vi "Main.vi"() -> ()   [LabVIEW 2019]
doc: "This template is for the Queued Message Handler design pattern.\n\nThe Event Handling Loop generates messages based on user interface actions.\n\nThe Message Handling Loop processes messages generated by the Event Handling Loop, or by other messages. The messages are string values, so new messages can be added easily to the Message Cases case structure in the Message Handling Loop. Each message cluster can also provide an optional value for Message Data, which is a variant that can be converted to whatever message-specific data is required."
uses:
  controls/UI Data.ctl
  C:/Program Files (x86)/National Instruments/LabVIEW 2019/examples/Instrument IO/Serial/support/Serial - Settings.ctl
  support/Message Queue/Enqueue Message (Single).vi
  support/Message Queue/Enqueue Message (Array).vi
  <instrlib>/Yokogawa WT300 Series/Public/Utility/Function/Create Function String (Voltage).vi
  <instrlib>/Yokogawa WT300 Series/Public/Data/Read Measurement (Normal).vi
  <instrlib>/Yokogawa WT300 Series/Public/Utility/Function/Create Function String (Current).vi
  <instrlib>/Yokogawa WT300 Series/Public/Utility/Function/Create Function String (Power).vi
  <instrlib>/Yokogawa WT300 Series/Public/Utility/Function/Create Function String (Integrate).vi
  <vilib>/Instr/_visa.llb/VISA Configure Serial Port (Instr).vi
  <vilib>/Utility/error.llb/Error Cluster From Error Code.vi
  <vilib>/ErrorRing/Error Ring.xnode
  support/Message Queue/Message Queue.lvlib
  support/User Event - Stop/User Event - Stop.lvlib
  <instrlib>/Yokogawa WT300 Series/Yokogawa WT300 Series.lvlib
  <instrlib>/Prodigit 331xF Series/Prodigit 331xF Series.lvlib
panel:
  in  "Tab Control":enum32{"General Setup", "Efficiency Test"}(tab)
  in  "AC Source Address":refnum<visa-resource-name>
  in  "Load Address":refnum<visa-resource-name>
  in  "Model Name":string
  in  "Switch":refnum<visa-resource-name>
  in  "PM Address":refnum<visa-resource-name>
  in  "Load":enum16{"ABC", "DEF", "GHI"}(ring)
  in  "Load(A)":dbl
  in  "Socket":enum16{"ABC", "DEF", "GHI"}(ring)
  in  "Input_Source[]":T1(array[ring])
  in  "Warm(s)":dbl
  out "Output_Load[]":dbl[](array[numeric])
  out "EFF":dbl format="%#_2f"
  out "P.F":dbl format="%#_2f"
  out "Counter":string
  out "V":dbl format="%#_5g"
  out "W":dbl format="%#_5g"
  out "A":dbl format="%#_5g"
  out "Function":string[](array[string])
  out "Measurement":dbl[](array[numeric])
  out "W":dbl format="%#_2f"
  out "A":dbl format="%#_2f"
  out "V":dbl format="%#_2f"
  out "Status":string
  in  "Do Something Else <Replace Me>":bool
  in  "Do Something <Replace Me>":bool
  in  "Exit":bool
  # "100%"
  # "75%"
  # "50%"
  # "25%"
  # "0%"
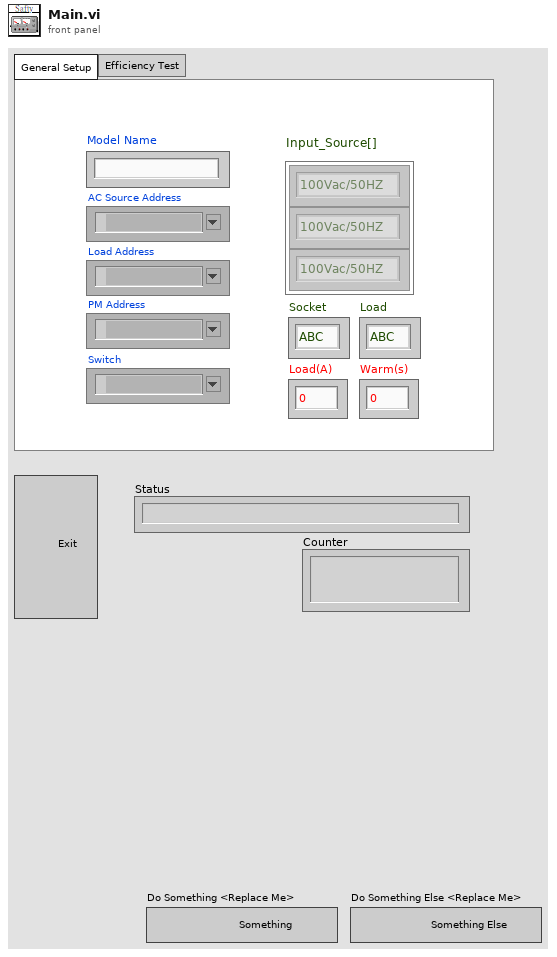
[diagram p1: front panel]
types:
  T1 = enum16{"100Vac/50HZ", "115Vac/60Hz", "230Vac/50Hz"}[]
  T2 = typedef "UI Data.ctl" = cluster{"Boolean <Replace Me>":bool, "Message":string, "Numeric <Replace Me>":dbl, "Do Something Ref":refnum<vi>, "Serial - Settings.ctlDo Something Else Ref":refnum<vi>, "Data Display Ref":refnum<vi>, "Exit Button Ref":refnum<vi>, "Model Name":string, "Input_Source[]":enum16{"100Vac/50HZ", "115Vac/60Hz", "230Vac/50Hz"}[], "RlyPort":refnum<visa-resource-name>, "ACSourcePara":cluster{"RangSelect":enum16{":SOUR:RANG LOW;", ":SOUR:RANG HIGH;", ":SOUR:RANG AUTO;"}, "Volt(V)":string, "Freq(Hz)":string, "OutpSlect":enum16{":SOUR:TURN OFF;", ":SOUR:TURN ON;"}, "TurnSlect":enum16{":SOUR:TURN OFF;", ":SOUR:TURN ON;"}}, "Step":cluster{"UI":string[], "PM":string[], "Load":string[]}, "PM Address":refnum<visa-resource-name>, "InputData":cluster{"V":dbl[], "A":dbl[], "W":dbl[], "P.F":dbl[], "EFF":dbl[], "Record":bool}, "LoadAddress":refnum<visa-resource-name>, "RLY":cluster{"Num":enum16{"AA", "01", "02", "03", "04", "05", "06", "07", "08", "09", "10", "11", "12", "13", "14", "15", "16", "17", "18", "19", "20", "21", "22", "23", "24"}, "ON/OFF":bool, "REST?":u16}, "AC Source Address":refnum<visa-resource-name>, "WarmUp Time":dbl, "Integrate Time":dbl, "Function":string[], "Measurement":dbl[], "SourceIndex":i32, "Socket":enum16{"ABC", "DEF", "GHI"}, "LoadSel":enum16{"ABC", "DEF", "GHI"}, "Load":cluster{"Current Level (F:Low)":u16, "OutputLoad[]":dbl[], "Index":i32, "Load (ON/Off)":bool, "Channel (0:Channel 1)":u16, "Value[]":cluster{"A":dbl[], "W":dbl[], "V":dbl[]}, "Record":bool}}
  T3 = typedef "Message Queue.lvlib/All Message Queues.ctl" = cluster{"UI":refnum<queue>, "PM":refnum<queue>, "Load":refnum<queue>}
  T4 = cluster{"Current Level (F:Low)":u16, "OutputLoad[]":dbl[], "Index":i32, "Load (ON/Off)":bool, "Channel (0:Channel 1)":u16, "Value[]":cluster{"A":dbl[], "W":dbl[], "V":dbl[]}, "Record":bool}
  T5 = cluster{"Current Level (F:Low)":u16, "OutputLoad[]":dbl[], "Index":i32, "Load (ON/Off)":bool, "Channel (0:Channel 1)":u16, "Value[]":cluster{"A":dbl[], "W":dbl[], "V":dbl[]}, "Record":bool}[]
  T6 = cluster{"V":dbl[], "A":dbl[], "W":dbl[], "P.F":dbl[], "EFF":dbl[], "Record":bool}
  T7 = typedef "Serial - Settings.ctl" = cluster{"baud rate":u32, "data bits":u16, "parity":enum16{"None", "Odd", "Even", "Mark", "Space"}, "stop bits":u16, "flow control":u16}
  T8 = enum16{":SOUR:RANG LOW;", ":SOUR:RANG HIGH;", ":SOUR:RANG AUTO;"}
  T9 = enum16{"SetRange", "SetVoltage", "SetFreq", "OUTP", "TurnOn"}
  T10 = enum16{"AA", "01", "02", "03", "04", "05", "06", "07", "08", "09", "10", "11", "12", "13", "14", "15", "16", "17", "18", "19", "20", "21", "22", "23", "24"}
  T11 = enum16{"100Vac/50HZ", "115Vac/60Hz", "230Vac/50Hz"}
  T12 = cluster{"RangSelect":enum16{":SOUR:RANG LOW;", ":SOUR:RANG HIGH;", ":SOUR:RANG AUTO;"}, "Volt(V)":string, "Freq(Hz)":string, "OutpSlect":enum16{":SOUR:TURN OFF;", ":SOUR:TURN ON;"}, "TurnSlect":enum16{":SOUR:TURN OFF;", ":SOUR:TURN ON;"}}
  T13 = cluster{"Num":enum16{"AA", "01", "02", "03", "04", "05", "06", "07", "08", "09", "10", "11", "12", "13", "14", "15", "16", "17", "18", "19", "20", "21", "22", "23", "24"}, "ON/OFF":bool, "REST?":u16}
  T14 = cluster{"V":dbl[], "A":dbl[], "W":dbl[], "P.F":dbl[], "EFF":dbl[], "Record":bool}[]
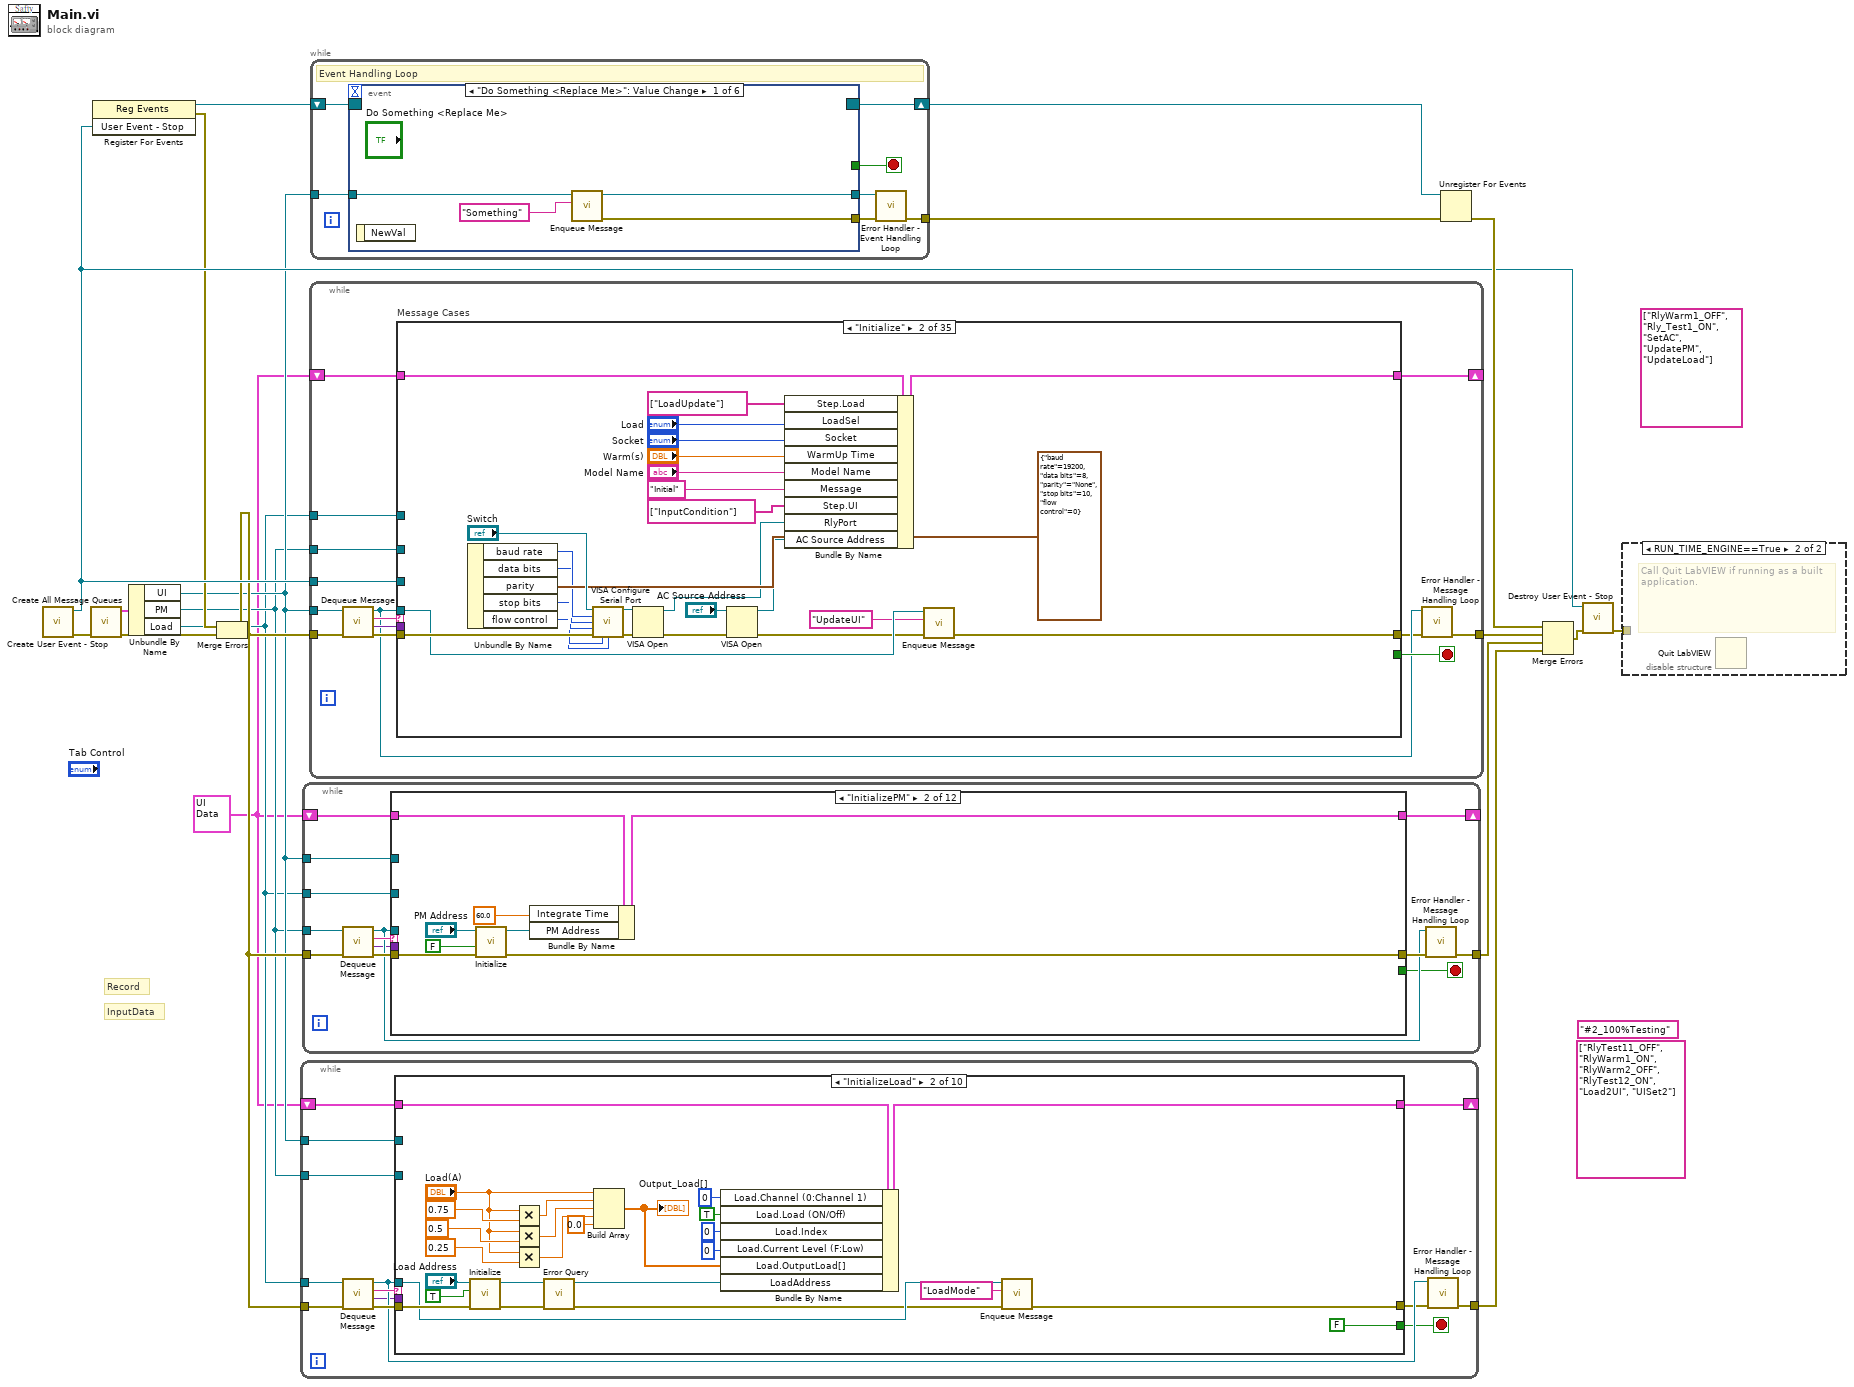
[diagram p0: block diagram]
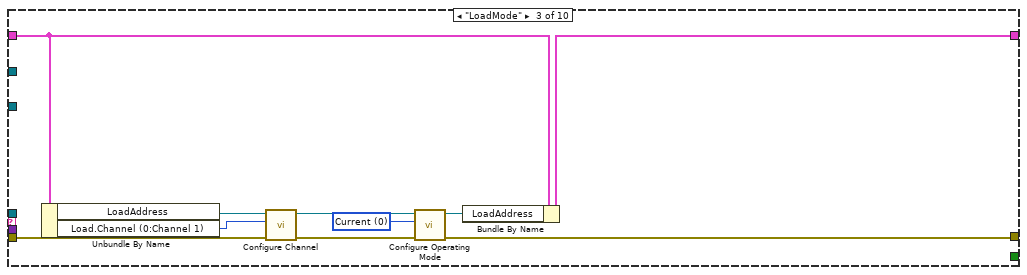
[diagram p3: hidden frame]
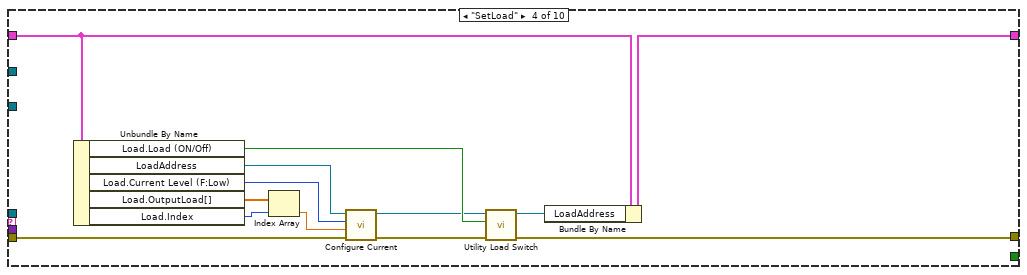
[diagram p4: hidden frame]
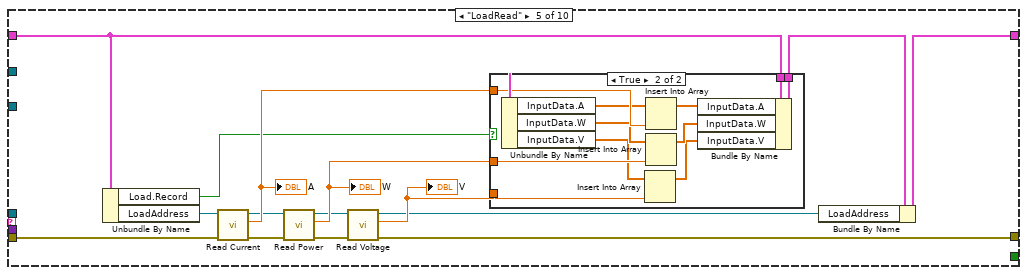
[diagram p5: hidden frame]
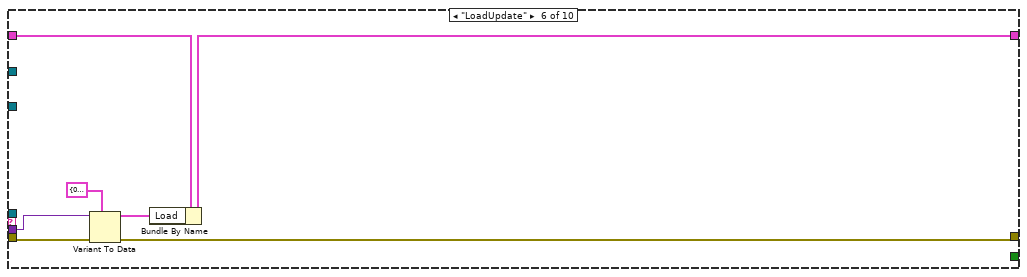
[diagram p7: hidden frame]
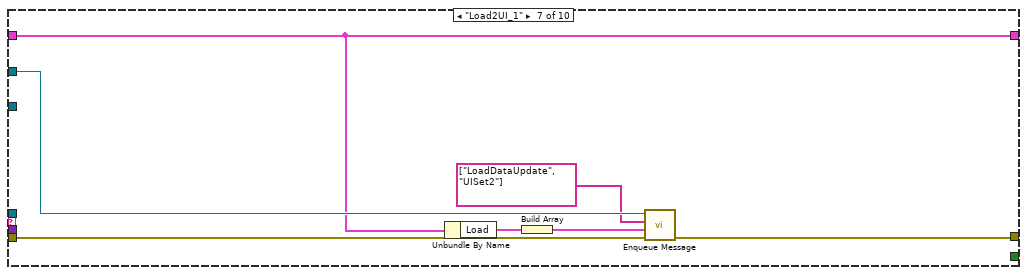
[diagram p8: hidden frame]
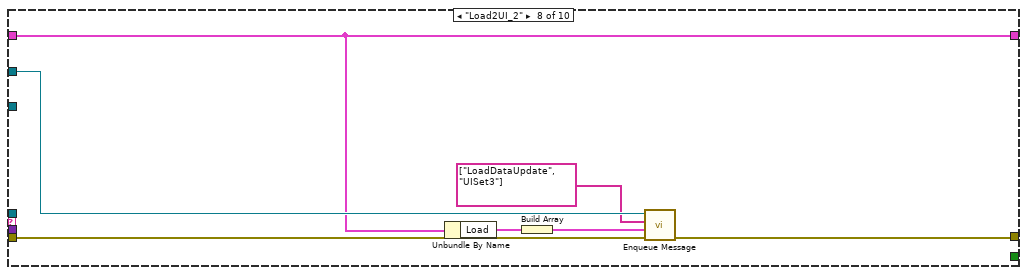
[diagram p9: hidden frame]
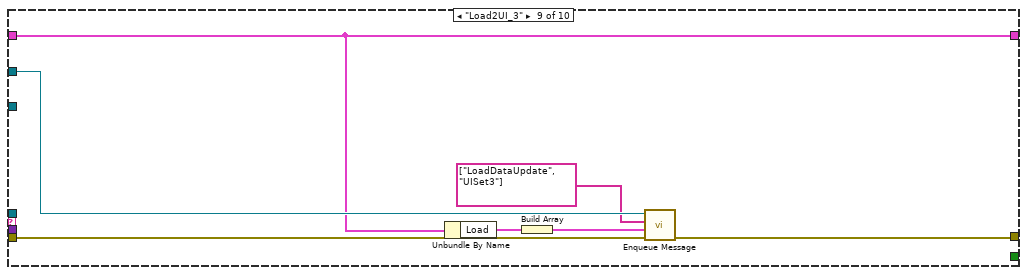
[diagram p10: hidden frame]
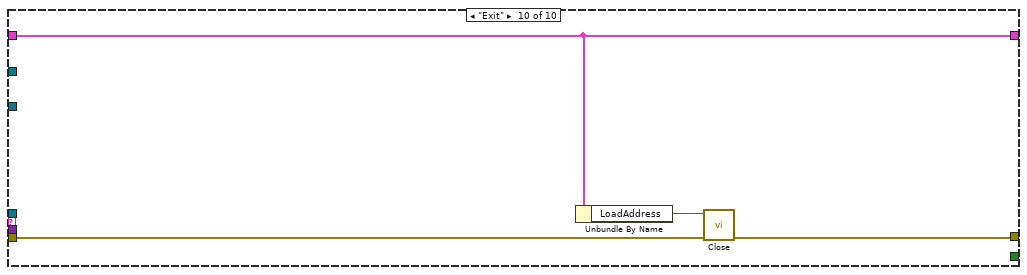
[diagram p11: hidden frame]
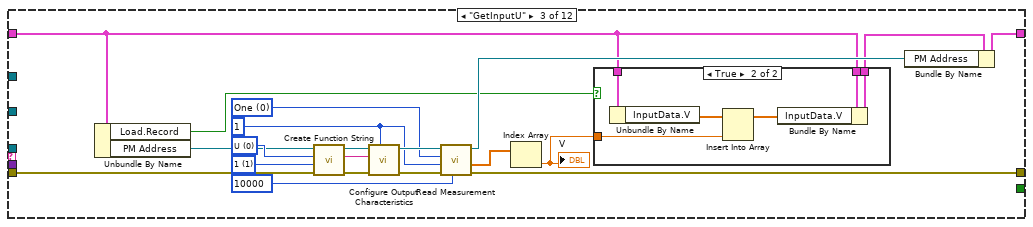
[diagram p13: hidden frame]
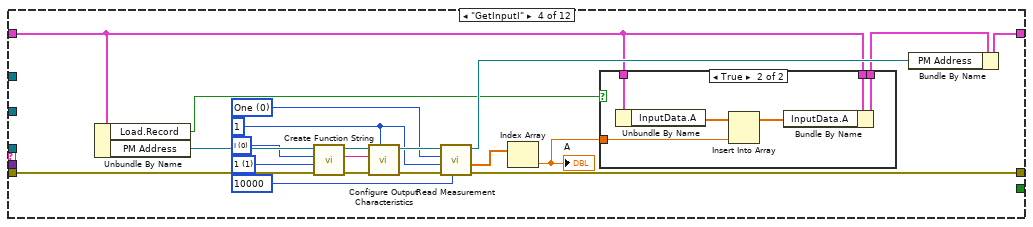
[diagram p15: hidden frame]
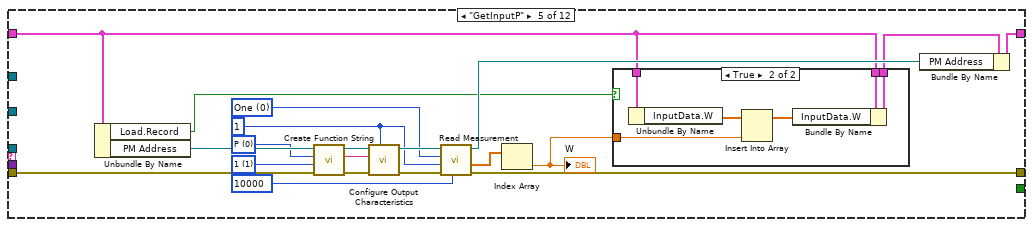
[diagram p17: hidden frame]
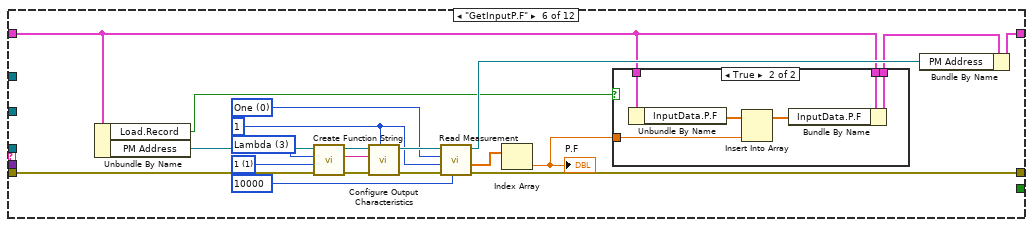
[diagram p19: hidden frame]
diagram:
  (unwired) string[] ["RlyWarm1_OFF", "Rly_Test1_ON", "SetAC", "UpdatePM", "UpdateLoad"] ("Step.UI")
  (unwired) "#2_100%Testing" ("Message")
  (unwired) string[] ["RlyTest11_OFF", "RlyWarm1_ON", "RlyWarm2_OFF", "RlyTest12_ON", "Load2UI", "UISet2"] ("Step.UI")
  w2 = T2 {"Boolean <Replace Me>"=FALSE, "Message"="", "Numeric <Replace Me>"=0.0, "Do Something Ref"=refnum, "Serial - Settings.ctlDo Something Else Ref"=refnum, "Data Display Ref"=refnum, "Exit Button Ref"=refnum, "Model Name"="", "Input_Source[]"=[enum."100Vac/50HZ", enum."115Vac/60Hz", enum."230Vac/50Hz"], "RlyPort"="COM1", "ACSourcePara"={"RangSelect"=enum.":SOUR:RANG AUTO;", "Volt(V)"="", "Freq(Hz)"="", "OutpSlect"=enum.":SOUR:TURN OFF;", "TurnSlect"=enum.":SOUR:TURN OFF;"}, "Step"={"UI"=[], "PM"=[], "Load"=[]}, "PM Address"="", "InputData"={"V"=[], "A"=[], "W"=[], "P.F"=[], "EFF"=[], "Record"=FALSE}, "LoadAddress"="", "RLY"={"Num"=enum."01", "ON/OFF"=FALSE, "REST?"=0}, "AC Source Address"="COM1", "WarmUp Time"=0.0, "Integrate Time"=0.0, "Function"=[], "Measurement"=[], "SourceIndex"=0, "Socket"=enum."ABC", "LoadSel"=enum."ABC", "Load"={"Current Level (F:Low)"=0, "OutputLoad[]"=[], "Index"=0, "Load (ON/Off)"=FALSE, "Channel (0:Channel 1)"=0, "Value[]"={"A"=[], "W"=[], "V"=[]}, "Record"=FALSE}} ("UI Data")
  # "InputData"
  # "Record"
  n1 = call "Create User Event - Stop.vi"() -> ("error out"=w16:errorcluster, "User Event - Stop"=w9:refnum<user-event>)  [unwired: 10 in]
  n2 = call "Create All Message Queues.vi"("error in (no error)"=w16) -> ("error out"=w19:errorcluster, "Message Queues out"=w18:T3)  [unwired: 9 in]
  n3 = register-events(w9) -> (reference out=w10:refnum<event-registration>, error out=w8:errorcluster)  [unwired: 2 in]
  n4 = Unbundle By Name(w18) -> ("UI"=w5:refnum<queue>, "PM"=w4:refnum<queue>, "Load"=w3:refnum<queue>)
  n5 = Merge Errors(w8, w19) -> (w6:errorcluster)
  n6 = while {
    tunnel: w3 -> [w32]
    tunnel: w6 -> [w31]
    shift-right: [w25] -> _
    shift-left: w2 -> [w26]
    tunnel: w5 -> [w23]
    tunnel: w4 -> [w22]
    tunnel: [w21] -> w1
    stop <- w27 stop-if-true
    n7 = call "Dequeue Message.vi"("error in (no error)"=w31, "Message Queue"=w32) -> ("error out"=w30:errorcluster, "Message Data"=w20:variant, "Message"=w29:string, "dup Message Queue"=w28:refnum<queue>)  [unwired: 6 in]
    n8 = case shown="\"InitializeLoad\"" w29 {
      tunnel: w30 -> [w34 w60 w62 w82 w92 w117 w123 w130 w137 w142]
      tunnel: w28 -> [_ w53 _ _ _ _ _ _ _ _]
      tunnel: [_ FALSE _ _ _ _ _ _ _ _] -> w27
      tunnel: w26 -> [w33 w58 w70 w75 w96 w115 w121 w128 w135 w139]
      tunnel: [w33 w57 w69 w73 w84 w114 w121 w128 w135 w139] -> w25
      tunnel: [w34 w54 w66 w77 w98 w113 w122 w129 w136 w141] -> w24
      tunnel: w23 -> [_ _ _ _ _ _ w124 w131 w138 _]
      tunnel: w22 -> [_ _ _ _ _ _ _ _ _ _]
      tunnel: w20 -> [_ _ _ _ _ w116 _ _ _ _]
      frame "WaitLoad", Default {
      }
      frame "InitializeLoad" {
        n9 = call <instrlib>:"Initialize.vi"("error in (no error)"=w60, "ID Query (True)"=TRUE, "VISA resource name"="Load Address") -> ("error out"=w39:errorcluster, "VISA resource name out"=w37:refnum<visa-resource-name>)  [unwired: 7 in]
        n10 = Multiply(x="Load(A)", y=0.75) -> (x*y=w46:dbl)
        n11 = Multiply(x="Load(A)", y=0.5) -> (x*y=w44:dbl)
        n12 = Multiply(x="Load(A)", y=0.25) -> (x*y=w43:dbl)
        n13 = call <instrlib>:"Error Query.vi"("error in (no error)"=w39, "VISA resource name"=w37) -> ("error out"=w38:errorcluster, "VISA resource name out"=w36:refnum<visa-resource-name>)  [unwired: 6 in, 2 out]
        n14 = Build Array("Load(A)", w46, w44, w43, 0.0 ("element")) -> (w41:dbl[])
        "Output_Load[]" <- w41
        n15 = Bundle By Name(cluster=w58, "Load.Channel (0:Channel 1)"=u16 0, "Load.Load (ON/Off)"=TRUE ("Load (F:Off)"), "Load.Index"=0, "Load.Current Level (F:Low)"=u16 0, "Load.OutputLoad[]"=w41, "LoadAddress"=w36) -> (w57:T2)
        n16 = call-poly "Enqueue Message.vi"("error in (no error)"=w38, "Message"="LoadMode", "Message Queue"=w53) -> ("error out"=w54:errorcluster)  [unwired: 7 in, 1 out]
      }
      frame "LoadMode" {
        w68 = 0 items=["Current", "Resistance", "Voltage", "Power"] ("Regulation Mode (0:Current)")
        n17 = Unbundle By Name(w70) -> ("LoadAddress"=w63:refnum<visa-resource-name>, "Load.Channel (0:Channel 1)"=w61:u16)
        n18 = call <instrlib>:"Configure Channel.vi"("error in (no error)"=w62, "Channel (0:Channel 1)"=w61, "VISA resource name"=w63) -> ("error out"=w65:errorcluster, "VISA resource name out"=w64:refnum<visa-resource-name>)  [unwired: 7 in]
        n19 = call <instrlib>:"Configure Operating Mode.vi"("error in (no error)"=w65, "Regulation Mode (0:Current)"=w68, "VISA resource name"=w64) -> ("error out"=w66:errorcluster, "VISA resource name out"=w67:refnum<visa-resource-name>)  [unwired: 7 in]
        n20 = Bundle By Name(cluster=w70, "LoadAddress"=w67) -> (w69:T2)
      }
      frame "SetLoad" {
        n21 = Unbundle By Name(w75) -> ("Load.Load (ON/Off)"=w76:bool, "LoadAddress"=w83:refnum<visa-resource-name>, "Load.Current Level (F:Low)"=w78:u16, "Load.OutputLoad[]"=w81:dbl[], "Load.Index"=w80:i32)
        n22 = Index Array(array=w81, index=w80) -> (element=w79:dbl)
        n23 = call <instrlib>:"Configure Current.vi"("error in (no error)"=w82, "Current (0.0 A)"=w79, "Current Level (F:Low)"=w78, "VISA resource name"=w83) -> ("error out"=w71:errorcluster, "VISA resource name out"=w72:refnum<visa-resource-name>)  [unwired: 6 in]
        n24 = call <instrlib>:"Utility Load Switch.vi"("error in (no error)"=w71, "Load (F:Off)"=w76, "VISA resource name"=w72) -> ("error out"=w77:errorcluster, "VISA resource name out"=w74:refnum<visa-resource-name>)  [unwired: 7 in]
        n25 = Bundle By Name(cluster=w75, "LoadAddress"=w74) -> (w73:T2)
      }
      frame "LoadRead" {
        n26 = Unbundle By Name(w96) -> ("Load.Record"=w87:bool, "LoadAddress"=w97:refnum<visa-resource-name>)
        n27 = call <instrlib>:"Read Current.vi"("error in (no error)"=w92, "VISA resource name"=w97) -> ("error out"=w89:errorcluster, "Current(A)"=w95:dbl, "VISA resource name out"=w88:refnum<visa-resource-name>)  [unwired: 7 in]
        "A" <- w95
        n28 = call <instrlib>:"Read Power.vi"("error in (no error)"=w89, "VISA resource name"=w88) -> ("error out"=w91:errorcluster, "Power(W)"=w94:dbl, "VISA resource name out"=w90:refnum<visa-resource-name>)  [unwired: 7 in]
        "W" <- w94
        n29 = call <instrlib>:"Read Voltage.vi"("error in (no error)"=w91, "VISA resource name"=w90) -> ("error out"=w98:errorcluster, "Voltage(V)"=w93:dbl, "VISA resource name out"=w86:refnum<visa-resource-name>)  [unwired: 7 in]
        "V" <- w93
        n30 = case shown="True" w87 {
          tunnel: w96 -> [w99 w110]
          tunnel: w95 -> [_ w109]
          tunnel: w94 -> [_ w108]
          tunnel: w93 -> [_ w107]
          tunnel: [w99 w100] -> w85
          frame False {
          }
          frame True {
            n31 = Unbundle By Name(w110) -> ("InputData.A"=w106:dbl[], "InputData.W"=w104:dbl[], "InputData.V"=w102:dbl[])
            n32 = Insert Into Array(array=w102, new element=w107) -> (w101:dbl[])  [unwired: 1 in]
            n33 = Insert Into Array(array=w106, new element=w109) -> (w105:dbl[])  [unwired: 1 in]
            n34 = Insert Into Array(array=w104, new element=w108) -> (w103:dbl[])  [unwired: 1 in]
            n35 = Bundle By Name(cluster=w110, "InputData.A"=w105, "InputData.W"=w103, "InputData.V"=w101) -> (w100:T2)
          }
        }
        n36 = Bundle By Name(cluster=w85, "LoadAddress"=w86) -> (w84:T2)
      }
      frame "LoadUpdate" {
        n37 = Variant To Data(error in=w117, type=T4 {"Current Level (F:Low)"=0, "OutputLoad[]"=[], "Index"=0, "Load (ON/Off)"=FALSE, "Channel (0:Channel 1)"=0, "Value[]"={"A"=[], "W"=[], "V"=[]}, "Record"=FALSE} ("Load"), Variant=w116) -> (data=w111:T4, error out=w113:errorcluster)
        n38 = Bundle By Name(cluster=w115, "Load"=w111) -> (w114:T2)
      }
      frame "Load2UI_1" {
        n39 = Unbundle By Name(w121) -> ("Load"=w120:T4)
        n40 = Build Array(w120) -> (w118:T5)
        n41 = call-poly "Enqueue Message.vi"("error in (no error)"=w123, "Message Data Array"=w118, "Message Array"=string[] ["LoadDataUpdate", "UISet2"], "Message Queue"=w124) -> ("error out"=w122:errorcluster)  [unwired: 6 in, 1 out]
      }
      frame "Load2UI_2" {
        n42 = Unbundle By Name(w128) -> ("Load"=w127:T4)
        n43 = Build Array(w127) -> (w125:T5)
        n44 = call-poly "Enqueue Message.vi"("error in (no error)"=w130, "Message Data Array"=w125, "Message Array"=string[] ["LoadDataUpdate", "UISet3"], "Message Queue"=w131) -> ("error out"=w129:errorcluster)  [unwired: 6 in, 1 out]
      }
      frame "Load2UI_3" {
        n45 = Unbundle By Name(w135) -> ("Load"=w134:T4)
        n46 = Build Array(w134) -> (w132:T5)
        n47 = call-poly "Enqueue Message.vi"("error in (no error)"=w137, "Message Data Array"=w132, "Message Array"=string[] ["LoadDataUpdate", "UISet3"], "Message Queue"=w138) -> ("error out"=w136:errorcluster)  [unwired: 6 in, 1 out]
      }
      frame "Exit" {
        n48 = Unbundle By Name(w139) -> ("LoadAddress"=w140:refnum<visa-resource-name>)
        n49 = call <instrlib>:"Close.vi"("error in (no error)"=w142, "VISA resource name"=w140) -> ("error out"=w141:errorcluster)  [unwired: 9 in]
      }
    }
    n50 = call "Error Handler - Message Handling Loop.vi"("error in (no error)"=w24, "Message Queue"=w28) -> ("dup error in"=w21:errorcluster)  [unwired: 8 in, 1 out]
  }
  n51 = while {
    tunnel: w4 -> [w155]
    tunnel: w6 -> [w154]
    tunnel: [w148] -> w7
    shift-right: [w150] -> _
    shift-left: w2 -> [w151]
    tunnel: w5 -> [w145]
    tunnel: w3 -> [w144]
    stop <- w146 stop-if-true
    n52 = call "Dequeue Message.vi"("error in (no error)"=w154, "Message Queue"=w155) -> ("error out"=w152:errorcluster, "Message Data"=w143:variant, "Message"=w153:string, "dup Message Queue"=w147:refnum<queue>)  [unwired: 6 in]
    n53 = case shown="\"InitializePM\"" w153 {
      tunnel: w147 -> [_ _ _ _ _ _ _ _ _ _ _ _]
      tunnel: w152 -> [w157 w162 w174 w202 w229 w256 w284 w336 w349 w357 w362 w368]
      tunnel: [w157 w165 w173 w201 w228 w255 w283 w324 w350 w352 w361 w369] -> w149
      tunnel: w151 -> [w156 w164 w167 w197 w224 w251 w279 w319 w347 w355 w360 w365]
      tunnel: [w156 w163 w170 w198 w225 w252 w280 w317 w347 w353 w360 w365] -> w150
      tunnel: [_ _ _ _ _ _ _ _ _ _ _ TRUE] -> w146
      tunnel: w145 -> [_ _ _ _ _ _ _ _ w351 _ w359 _]
      tunnel: w144 -> [_ _ _ _ _ _ _ _ _ _ _ _]
      tunnel: w143 -> [_ _ _ _ _ _ _ _ _ w358 _ _]
      frame "WaitPM", Default {
      }
      frame "InitializePM" {
        n54 = call <instrlib>:"Initialize.vi"("error in (no error)"=w162, "Reset (True)"=FALSE, "VISA resource name"="PM Address") -> ("error out"=w165:errorcluster, "VISA resource name out"=w159:refnum<visa-resource-name>)  [unwired: 7 in]
        n55 = Bundle By Name(cluster=w164, "Integrate Time"=60.0, "PM Address"=w159) -> (w163:T2)
      }
      frame "GetInputU" {
        w176 = 1 items=["1"=1, "2"=2, "3"=3, "Sigma A"=4] ("Element (1: 1)")
        w175 = 0 items=["U", "UPPeak", "UMPeak"] ("Function (0: U)")
        w178 = 1 ("Item (1)")
        w177 = 0 items=["One", "Plural"] ("Measure Item")
        n56 = Unbundle By Name(w167) -> ("Load.Record"=w169:bool, "PM Address"=w172:refnum<visa-resource-name>)
        n57 = call-poly <instrlib>:"Create Function String.vi"("error in (no error)"=w174, "Element (1: 1)"=w176, "Function (0: U)"=w175, "VISA resource name"=w172) -> ("error out"=w183:errorcluster, "Function String"=w184:string, "VISA resource name out"=w182:refnum<visa-resource-name>)  [unwired: 5 in]
        n58 = call <instrlib>:"Configure Output Characteristics.vi"("Item (1)"=w178, "error in (no error)"=w183, "Function (Empty)"=w184, "VISA resource name"=w182) -> ("error out"=w181:errorcluster, "VISA resource name out"=w180:refnum<visa-resource-name>)  [unwired: 6 in]
        n59 = call-poly <instrlib>:"Read Measurement.vi"("Timeout (10000 ms)"=10000, "error in (no error)"=w181, "Number of Item (15)"=w178, "Measure Item (1: Plural)"=w177, "VISA resource name"=w180) -> ("error out"=w173:errorcluster, "Measurement"=w185:dbl[], "VISA resource name out"=w171:refnum<visa-resource-name>)  [unwired: 3 in, 1 out]
        n60 = Index Array(array=w185) -> (element=w168:dbl)  [unwired: 1 in]
        "V" <- w168
        n61 = case shown="True" w169 {
          tunnel: w167 -> [_ w192]
          tunnel: w168 -> [_ w190]
          tunnel: w167 -> [w186 w189]
          tunnel: [w186 w187] -> w166
          frame False {
          }
          frame True {
            n62 = Unbundle By Name(w192) -> ("InputData.V"=w191:dbl[])
            n63 = Insert Into Array(array=w191, new element=w190) -> (w188:dbl[])  [unwired: 1 in]
            n64 = Bundle By Name(cluster=w189, "InputData.V"=w188) -> (w187:T2)
          }
        }
        n65 = Bundle By Name(cluster=w166, "PM Address"=w171) -> (w170:T2)
      }
      frame "GetInputI" {
        w193 = 0 items=["I", "IPPeak", "IMPeak"] ("Function (0: I)")
        w203 = 1 items=["1"=1, "2"=2, "3"=3, "Sigma A"=4] ("Element (1: 1)")
        w205 = 1 ("Item (1)")
        w204 = 0 items=["One", "Plural"] ("Measure Item")
        n66 = Unbundle By Name(w197) -> ("Load.Record"=w194:bool, "PM Address"=w200:refnum<visa-resource-name>)
        n67 = call-poly <instrlib>:"Create Function String.vi"("error in (no error)"=w202, "Element (1: 1)"=w203, "Function (0: I)"=w193, "VISA resource name"=w200) -> ("error out"=w210:errorcluster, "Function String"=w211:string, "VISA resource name out"=w209:refnum<visa-resource-name>)  [unwired: 5 in]
        n68 = call <instrlib>:"Configure Output Characteristics.vi"("Item (1)"=w205, "error in (no error)"=w210, "Function (Empty)"=w211, "VISA resource name"=w209) -> ("error out"=w208:errorcluster, "VISA resource name out"=w207:refnum<visa-resource-name>)  [unwired: 6 in]
        n69 = call-poly <instrlib>:"Read Measurement.vi"("Timeout (10000 ms)"=10000, "error in (no error)"=w208, "Number of Item (15)"=w205, "Measure Item (1: Plural)"=w204, "VISA resource name"=w207) -> ("error out"=w201:errorcluster, "Measurement"=w212:dbl[], "VISA resource name out"=w199:refnum<visa-resource-name>)  [unwired: 3 in, 1 out]
        n70 = Index Array(array=w212) -> (element=w195:dbl)  [unwired: 1 in]
        "A" <- w195
        n71 = case shown="True" w194 {
          tunnel: w197 -> [_ w219]
          tunnel: w195 -> [_ w217]
          tunnel: w197 -> [w213 w216]
          tunnel: [w213 w214] -> w196
          frame False {
          }
          frame True {
            n72 = Unbundle By Name(w219) -> ("InputData.A"=w218:dbl[])
            n73 = Insert Into Array(array=w218, new element=w217) -> (w215:dbl[])  [unwired: 1 in]
            n74 = Bundle By Name(cluster=w216, "InputData.A"=w215) -> (w214:T2)
          }
        }
        n75 = Bundle By Name(cluster=w196, "PM Address"=w199) -> (w198:T2)
      }
      frame "GetInputP" {
        w220 = 0 items=["P", "S", "Q", "Lambda", "Phi", "P+peak", "P-peak"] ("Function (0: P)")
        w230 = 1 items=["1"=1, "2"=2, "3"=3, "Sigma A"=4] ("Element (1: 1)")
        w232 = 1 ("Item (1)")
        w231 = 0 items=["One", "Plural"] ("Measure Item")
        n76 = Unbundle By Name(w224) -> ("Load.Record"=w221:bool, "PM Address"=w227:refnum<visa-resource-name>)
        n77 = call-poly <instrlib>:"Create Function String.vi"("error in (no error)"=w229, "Element (1: 1)"=w230, "Function (0: P)"=w220, "VISA resource name"=w227) -> ("error out"=w237:errorcluster, "Function String"=w238:string, "VISA resource name out"=w236:refnum<visa-resource-name>)  [unwired: 5 in]
        n78 = call <instrlib>:"Configure Output Characteristics.vi"("Item (1)"=w232, "error in (no error)"=w237, "Function (Empty)"=w238, "VISA resource name"=w236) -> ("error out"=w235:errorcluster, "VISA resource name out"=w234:refnum<visa-resource-name>)  [unwired: 6 in]
        n79 = call-poly <instrlib>:"Read Measurement.vi"("Timeout (10000 ms)"=10000, "error in (no error)"=w235, "Number of Item (15)"=w232, "Measure Item (1: Plural)"=w231, "VISA resource name"=w234) -> ("error out"=w228:errorcluster, "Measurement"=w239:dbl[], "VISA resource name out"=w226:refnum<visa-resource-name>)  [unwired: 3 in, 1 out]
        n80 = Index Array(array=w239) -> (element=w222:dbl)  [unwired: 1 in]
        "W" <- w222
        n81 = case shown="True" w221 {
          tunnel: w224 -> [_ w246]
          tunnel: w222 -> [_ w244]
          tunnel: w224 -> [w240 w243]
          tunnel: [w240 w241] -> w223
          frame False {
          }
          frame True {
            n82 = Unbundle By Name(w246) -> ("InputData.W"=w245:dbl[])
            n83 = Insert Into Array(array=w245, new element=w244) -> (w242:dbl[])  [unwired: 1 in]
            n84 = Bundle By Name(cluster=w243, "InputData.W"=w242) -> (w241:T2)
          }
        }
        n85 = Bundle By Name(cluster=w223, "PM Address"=w226) -> (w225:T2)
      }
      frame "GetInputP.F" {
        w247 = 3 items=["P", "S", "Q", "Lambda", "Phi", "P+peak", "P-peak"] ("Function (0: P)")
        w257 = 1 items=["1"=1, "2"=2, "3"=3, "Sigma A"=4] ("Element (1: 1)")
        w259 = 1 ("Item (1)")
        w258 = 0 items=["One", "Plural"] ("Measure Item")
        n86 = Unbundle By Name(w251) -> ("Load.Record"=w248:bool, "PM Address"=w254:refnum<visa-resource-name>)
        n87 = call-poly <instrlib>:"Create Function String.vi"("error in (no error)"=w256, "Element (1: 1)"=w257, "Function (0: P)"=w247, "VISA resource name"=w254) -> ("error out"=w264:errorcluster, "Function String"=w265:string, "VISA resource name out"=w263:refnum<visa-resource-name>)  [unwired: 5 in]
        n88 = call <instrlib>:"Configure Output Characteristics.vi"("Item (1)"=w259, "error in (no error)"=w264, "Function (Empty)"=w265, "VISA resource name"=w263) -> ("error out"=w262:errorcluster, "VISA resource name out"=w261:refnum<visa-resource-name>)  [unwired: 6 in]
        n89 = call-poly <instrlib>:"Read Measurement.vi"("Timeout (10000 ms)"=10000, "error in (no error)"=w262, "Number of Item (15)"=w259, "Measure Item (1: Plural)"=w258, "VISA resource name"=w261) -> ("error out"=w255:errorcluster, "Measurement"=w266:dbl[], "VISA resource name out"=w253:refnum<visa-resource-name>)  [unwired: 3 in, 1 out]
        n90 = Index Array(array=w266) -> (element=w249:dbl)  [unwired: 1 in]
        "P.F" <- w249
        n91 = case shown="True" w248 {
          tunnel: w251 -> [_ w273]
          tunnel: w249 -> [_ w271]
          tunnel: w251 -> [w267 w270]
          tunnel: [w267 w268] -> w250
          frame False {
          }
          frame True {
            n92 = Unbundle By Name(w273) -> ("InputData.P.F"=w272:dbl[])
            n93 = Insert Into Array(array=w272, new element=w271) -> (w269:dbl[])  [unwired: 1 in]
            n94 = Bundle By Name(cluster=w270, "InputData.P.F"=w269) -> (w268:T2)
          }
        }
        n95 = Bundle By Name(cluster=w250, "PM Address"=w253) -> (w252:T2)
      }
      frame "GetEFF" {
        w274 = 1 items=["1"=1, "2"=2, "3"=3, "Sigma A"=4] ("Element (1: 1)")
        w275 = 7 items=["Time", "WP", "WP+", "WP-", "q", "q+", "q-", "Math"] ("Function (0: Time)")
        w286 = 1 ("Item (1)")
        w285 = 0 items=["One", "Plural"] ("Measure Item")
        n96 = Unbundle By Name(w279) -> ("Load.Record"=w276:bool, "PM Address"=w282:refnum<visa-resource-name>)
        n97 = call-poly <instrlib>:"Create Function String.vi"("error in (no error)"=w284, "Element (1: 1)"=w274, "Function (0: Time)"=w275, "VISA resource name"=w282) -> ("error out"=w291:errorcluster, "Function String"=w292:string, "VISA resource name out"=w290:refnum<visa-resource-name>)  [unwired: 5 in]
        n98 = call <instrlib>:"Configure Output Characteristics.vi"("Item (1)"=w286, "error in (no error)"=w291, "Function (Empty)"=w292, "VISA resource name"=w290) -> ("error out"=w289:errorcluster, "VISA resource name out"=w288:refnum<visa-resource-name>)  [unwired: 6 in]
        n99 = call-poly <instrlib>:"Read Measurement.vi"("Timeout (10000 ms)"=10000, "error in (no error)"=w289, "Number of Item (15)"=w286, "Measure Item (1: Plural)"=w285, "VISA resource name"=w288) -> ("error out"=w283:errorcluster, "Measurement"=w293:dbl[], "VISA resource name out"=w281:refnum<visa-resource-name>)  [unwired: 3 in, 1 out]
        n100 = Index Array(array=w293) -> (element=w277:dbl)  [unwired: 1 in]
        "EFF" <- w277
        n101 = case shown="True" w276 {
          tunnel: w279 -> [_ w300]
          tunnel: w277 -> [_ w298]
          tunnel: w279 -> [w294 w297]
          tunnel: [w294 w295] -> w278
          frame False {
          }
          frame True {
            n102 = Unbundle By Name(w300) -> ("InputData.EFF"=w299:dbl[])
            n103 = Insert Into Array(array=w299, new element=w298) -> (w296:dbl[])  [unwired: 1 in]
            n104 = Bundle By Name(cluster=w297, "InputData.EFF"=w296) -> (w295:T2)
          }
        }
        n105 = Bundle By Name(cluster=w278, "PM Address"=w281) -> (w280:T2)
      }
      frame "Integrate" {
        w309 = 1 items=["1"=1, "2"=2, "3"=3, "Sigma A"=4] ("Element (1: 1)")
        w308 = 1 ("Item (1)")
        w310 = 7 items=["Time", "WP", "WP+", "WP-", "q", "q+", "q-", "Math"] ("Function (0: Time)")
        w322 = 0.5 items=["100m"=0.1, "250m"=0.25, "500m"=0.5, "1"=1.0, "2"=2.0, "5"=5.0] ("Update Rate (500m s)")
        n106 = Unbundle By Name(w319) -> ("InputData.EFF"=w304:dbl[], "Integrate Time"=w316:dbl, "PM Address"=w335:refnum<visa-resource-name>)
        n107 = call <instrlib>:"Configure Sample Update Rate.vi"("error in (no error)"=w336, "Update Rate (500m s)"=w322, "VISA resource name"=w335) -> ("error out"=w334:errorcluster, "VISA resource name out"=w333:refnum<visa-resource-name>)  [unwired: 7 in]
        n108 = call-poly <instrlib>:"Create Function String.vi"("error in (no error)"=w334, "Element (1: 1)"=w309, "Function (0: Time)"=w310, "VISA resource name"=w333) -> ("error out"=w311:errorcluster, "Function String"=w313:string, "VISA resource name out"=w312:refnum<visa-resource-name>)  [unwired: 5 in]
        n109 = To Unsigned Long Integer(number=w322) -> (unsigned 32bit integer=w307:u32)
        n110 = call <instrlib>:"Configure Output Characteristics.vi"("Item (1)"=w308, "error in (no error)"=w311, "Function (Empty)"=w313, "VISA resource name"=w312) -> ("error out"=w331:errorcluster, "VISA resource name out"=w332:refnum<visa-resource-name>)  [unwired: 6 in]
        n111 = Multiply(x=u32 1000, y=w307) -> (x*y=w321:u32)
        n112 = call <instrlib>:"Integrate Start.vi"("error in (no error)"=w331, "VISA resource name"=w332) -> ("error out"=w330:errorcluster, "VISA resource name out"=w329:refnum<visa-resource-name>)  [unwired: 8 in]
        n113 = To Long Integer(number=w316) -> (32bit integer=w315:i32)
        n114 = for {
          N: w315 -> [_]
          tunnel: w330 -> [w346]
          tunnel: w329 -> [w344]
          tunnel: w308 -> [w343]
          tunnel: [w342] -> w325
          tunnel: [w341] -> w326
          tunnel: w321 -> [w337]
          tunnel: 10000 ("Timeout (10000 ms)") -> [w340]
          tunnel: [w339] -> w301
          tunnel: [w338] -> w314
          w345 = 1 items=["One", "Plural"] ("Measure Item (1: Plural)")
          n115 = Wait Until Next ms Multiple(millisecond multiple=w337) -> ()  [unwired: 1 out]
          n116 = call-poly <instrlib>:"Read Measurement.vi"("Timeout (10000 ms)"=w340, "error in (no error)"=w346, "Number of Item (15)"=w343, "Measure Item (1: Plural)"=w345, "VISA resource name"=w344) -> ("error out"=w341:errorcluster, "Measurement"=w339:dbl[], "Function"=w338:string[], "VISA resource name out"=w342:refnum<visa-resource-name>)  [unwired: 3 in]
        }
        "Function" <- w314
        "Measurement" <- w301
        n117 = call <instrlib>:"Integrate Stop.vi"("error in (no error)"=w326, "VISA resource name"=w325) -> ("error out"=w327:errorcluster, "VISA resource name out"=w328:refnum<visa-resource-name>)  [unwired: 8 in]
        n118 = call <instrlib>:"Integrate Reset.vi"("error in (no error)"=w327, "VISA resource name"=w328) -> ("error out"=w324:errorcluster, "VISA resource name out"=w318:refnum<visa-resource-name>)  [unwired: 8 in]
        n119 = Array Size(array=w301) -> (size(s)=w306:i32)
        n120 = Decrement(x=w306) -> (x-1=w303:i32)
        n121 = Index Array(array=w301, index=w303) -> (element=w302:dbl)
        n122 = Insert Into Array(array=w304, new element=w302) -> (w305:dbl[])  [unwired: 1 in]
        n123 = Bundle By Name(cluster=w319, "InputData.EFF"=w305, "Function"=w314, "Measurement"=w301, "PM Address"=w318) -> (w317:T2)
      }
      frame "RlySet1" {
        n124 = call-poly "Enqueue Message.vi"("error in (no error)"=w349, "Message"="BurnIn", "Message Queue"=w351) -> ("error out"=w350:errorcluster)  [unwired: 7 in, 1 out]
      }
      frame "PMUpdate" {
        n125 = Variant To Data(error in=w357, type=T6 {"V"=[], "A"=[], "W"=[], "P.F"=[], "EFF"=[], "Record"=FALSE} ("InputData"), Variant=w358) -> (data=w354:T6, error out=w352:errorcluster)
        n126 = Bundle By Name(cluster=w355, "InputData"=w354) -> (w353:T2)
      }
      frame "PM2UI" {
        n127 = Unbundle By Name(w360) -> ("InputData"=w363:T6)
        n128 = call-poly "Enqueue Message.vi"("error in (no error)"=w362, "Message Data"=w363, "Message"="PMDataUpdate", "Message Queue"=w359) -> ("error out"=w361:errorcluster)  [unwired: 6 in, 1 out]
      }
      frame "Exit" {
        n129 = Unbundle By Name(w365) -> ("PM Address"=w367:refnum<visa-resource-name>)
        n130 = call <instrlib>:"Close.vi"("error in (no error)"=w368, "VISA resource name"=w367) -> ("error out"=w369:errorcluster)  [unwired: 9 in]
      }
    }
    n131 = call "Error Handler - Message Handling Loop.vi"("error in (no error)"=w149, "Message Queue"=w147) -> ("dup error in"=w148:errorcluster)  [unwired: 8 in, 1 out]
  }
  n132 = while {
    tunnel: w5 -> [w375]
    shift-right: [w382] -> _
    shift-left: w2 -> [w383]
    tunnel: w9 -> [w380]
    tunnel: w6 -> [w379]
    tunnel: [w373] -> w17
    tunnel: w4 -> [w371]
    tunnel: w3 -> [w370]
    stop <- w381 stop-if-true
    # "Message Handling Loop"
    n133 = call "Dequeue Message.vi"("error in (no error)"=w379, "Message Queue"=w375) -> ("error out"=w378:errorcluster, "Message Data"=w376:variant, "Message"=w377:string, "dup Message Queue"=w374:refnum<queue>)  [unwired: 6 in]
    n134 = case "Message Cases" shown="\"Initialize\"" w377 {
      selector: w377 -> [_ _ _ _ _ _ _ _ _ _ _ _ _ _ _ _ _ _ _ _ _ _ _ _ _ _ _ _ _ _ _ _ _ _ w935]
      tunnel: w374 -> [_ w405 w425 w433 w440 _ _ _ _ _ _ _ _ _ _ _ _ _ _ _ _ w821 w836 w851 w868 _ _ _ _ _ _ w916 _ w934 _]
      tunnel: w378 -> [w385 w409 w426 w435 w443 w480 w493 w510 w533 w556 w579 w602 w625 w648 w671 w694 w717 w740 w763 w786 w809 w823 w838 w853 w867 w875 w882 w888 w895 w899 w913 w920 w923 w927 _]
      tunnel: [w385 w400 w422 w434 w442 w462 w486 w499 w522 w545 w568 w591 w614 w637 w660 w683 w706 w729 w752 w775 w798 w822 w837 w852 w863 w872 w879 w887 w894 w898 w907 w918 w921 w930 w936] -> w372
      tunnel: w383 -> [w384 w404 w427 w437 w451 w461 w482 w506 w529 w552 w575 w598 w621 w644 w667 w690 w713 w736 w759 w782 w805 w832 w847 w862 w866 w871 w876 w885 w892 w906 w912 w919 w922 w933 w937]
      tunnel: [w384 w399 w414 w436 w450 w479 w487 w503 w526 w549 w572 w595 w618 w641 w664 w687 w710 w733 w756 w779 w802 w825 w840 w855 w866 w871 w876 w884 w891 w906 w912 w919 w922 w933 w937] -> w382
      tunnel: [_ _ _ _ _ _ _ _ _ _ _ _ _ _ _ _ _ _ _ _ _ _ _ _ _ _ _ _ _ _ _ _ _ TRUE _] -> w381
      tunnel: w376 -> [_ _ _ _ _ _ _ _ _ _ _ _ _ _ _ _ _ _ _ _ _ _ _ _ _ _ _ w886 w893 _ w911 _ _ w924 _]
      tunnel: w380 -> [_ _ _ _ _ _ _ _ _ _ _ _ _ _ _ _ _ _ _ _ _ _ _ _ _ _ _ _ _ _ _ _ _ w929 _]
      tunnel: w371 -> [_ _ _ _ _ _ _ _ _ _ _ _ _ _ _ _ _ _ _ _ _ _ _ _ _ w873 _ _ _ _ _ _ _ _ _]
      tunnel: w370 -> [_ _ _ _ _ _ _ _ _ _ _ _ _ _ _ _ _ _ _ _ _ _ _ _ _ _ w880 _ _ _ _ _ _ _ _]
      frame "WaitUI", Default {
      }
      frame "Initialize" {
        # "Initialize - All initialization work should take place in this message, since other loops can potentially enqueue messages that execute immediately after this one."
        n135 = Unbundle By Name(T7 {"baud rate"=19200, "data bits"=8, "parity"=enum."None", "stop bits"=10, "flow control"=0} ("Serial Settings")) -> ("baud rate"=w391:u32, "data bits"=w390:u16, "parity"=w389:enum16{"None", "Odd", "Even", "Mark", "Space"}, "stop bits"=w388:u16, "flow control"=w387:u16)
        n136 = call-poly "VISA Configure Serial Port"("VISA resource name"="Switch", "baud rate (9600)"=w391, "data bits (8)"=w390, "parity (0:none)"=w389, "error in (no error)"=w409, "stop bits (10: 1 bit)"=w388, "flow control (0:none)"=w387) -> ("VISA resource name out"=w393:refnum<visa-resource-name>, "error out"=w394:errorcluster)  [unwired: 2 in, 5 out]
        n137 = VISA Open(error in (no error)=w394, VISA resource name=w393) -> (VISA resource name=w402:refnum<visa-resource-name>, error out=w392:errorcluster)  [unwired: 3 in]
        n138 = VISA Open(error in (no error)=w392, VISA resource name="AC Source Address") -> (VISA resource name=w403:refnum<visa-resource-name>, error out=w400:errorcluster)  [unwired: 3 in]
        n139 = Bundle By Name(cluster=w404, "Step.Load"=string[] ["LoadUpdate"], "LoadSel"="Load", "Socket"="Socket", "WarmUp Time"="Warm(s)", "Model Name"="Model Name", "Message"="Initial" ("Initial Message"), "Step.UI"=string[] ["InputCondition"], "RlyPort"=w402, "AC Source Address"=w403) -> (w399:T2)
        n140 = call-poly "Enqueue Message.vi"("Message"="UpdateUI", "Message Queue"=w405) -> ()  [unwired: 8 in, 2 out]
      }
      frame "InputCondition" {
        # "Something - Replace this message with functionality for your own application."
        n141 = Bundle By Name(cluster=w427, "Message"="Check Input & Output", "Input_Source[]"="Input_Source[]", "ACSourcePara.RangSelect"=T8.":SOUR:RANG AUTO;", "ACSourcePara.OutpSlect"=enum16{":SOUR:TURN OFF;", ":SOUR:TURN ON;"}.":SOUR:TURN ON;", "ACSourcePara.TurnSlect"=enum16{":SOUR:TURN OFF;", ":SOUR:TURN ON;"}.":SOUR:TURN ON;", "SourceIndex"=0, "Step.UI"=string[] ["UpdatePM", "UpdateLoad"]) -> (w418:T2)
        n142 = Bundle By Name(cluster=w418, "Step.PM"=string[] ["GetInputU", "GetInputI", "GetInputP", "GetInputP.F", "GetEFF", "RlySet1"] ("StepName")) -> (w417:T2)
        n143 = Bundle By Name(cluster=w417, "Step.Load"=string[] ["SetLoad ", "LoadRead"], "Load.Load (ON/Off)"=TRUE ("Load (F:Off)")) -> (w415:T2)
        n144 = Bundle By Name(cluster=w415, "Load.Record"=FALSE ("Record")) -> (w414:T2)
        n145 = call-poly "Enqueue Message.vi"("error in (no error)"=w426, "Message Array"=string[] ["SetAC", "RlyInit", "RlyTest1_ON", "RlyLoad_ON", "UpdateUI"] ("Message"), "Message Queue"=w425) -> ("error out"=w422:errorcluster)  [unwired: 7 in, 1 out]
      }
      frame "BurnIn" {
        n146 = call-poly "Enqueue Message.vi"("error in (no error)"=w435, "Message Array"=string[] ["RlyTest1_OFF", "RlyWarm1_ON", "UpdateUI"] ("Step.UI"), "Message Queue"=w433) -> ("error out"=w434:errorcluster)  [unwired: 7 in, 1 out]
        n147 = Bundle By Name(cluster=w437, "Message"="Burn 30 mins", "Step.UI"=string[] ["Counter", "UISet1"]) -> (w436:T2)
      }
      frame "SetAC" {
        n148 = Unbundle By Name(w451) -> ("Input_Source[]"=w449:T1, "SourceIndex"=w447:i32)
        n149 = Index Array(array=w449, index=w447) -> (element=w454:T11)
        n150 = Array Size(array=w449) -> (size(s)=w448:i32)
        n151 = case shown="\"230Vac/50Hz\"" w454 {
          tunnel: ["50" "60" "50"] -> w452
          tunnel: ["100" "115" "230"] -> w453
          frame "100Vac/50HZ", Default {
          }
          frame "115Vac/60Hz" {
          }
          frame "230Vac/50Hz" {
          }
        }
        n152 = Greater?(x=w447, y=w448) -> (0:w446:bool)
        n153 = Bundle By Name(cluster=w451, "ACSourcePara.Volt(V)"=w453, "ACSourcePara.Freq(Hz)"=w452) -> (w450:T2)
        n154 = Select(t="Report", s=w446, f="PWON") -> (s? t:f=w441:string)
        n155 = call-poly "Enqueue Message.vi"("error in (no error)"=w443, "Message"=w441, "Message Queue"=w440) -> ("error out"=w442:errorcluster)  [unwired: 7 in, 1 out]
      }
      frame "PWON" {
        n156 = Unbundle By Name(w461) -> ("AC Source Address"=w478:refnum<visa-resource-name>, "ACSourcePara"=w464:T12)
        n157 = call "AC_Source_VISA.vi"("error_in"=w480, "Parameter"=w464, "Mode"=T9."SetRange", "VISA_in"=w478) -> ("error_out"=w475:errorcluster, "VISA_out"=w476:refnum<visa-resource-name>)  [unwired: 1 in, 1 out]
        n158 = call "AC_Source_VISA.vi"("error_in"=w475, "Parameter"=w464, "Mode"=T9."SetVoltage", "VISA_in"=w476) -> ("error_out"=w473:errorcluster, "VISA_out"=w472:refnum<visa-resource-name>)  [unwired: 1 in, 1 out]
        n159 = call "AC_Source_VISA.vi"("error_in"=w473, "Parameter"=w464, "Mode"=T9."SetFreq", "VISA_in"=w472) -> ("error_out"=w470:errorcluster, "VISA_out"=w469:refnum<visa-resource-name>)  [unwired: 1 in, 1 out]
        n160 = call "AC_Source_VISA.vi"("error_in"=w470, "Parameter"=w464, "Mode"=T9."OUTP", "VISA_in"=w469) -> ("error_out"=w467:errorcluster, "VISA_out"=w466:refnum<visa-resource-name>)  [unwired: 1 in, 1 out]
        n161 = call "AC_Source_VISA.vi"("error_in"=w467, "Parameter"=w464, "Mode"=T9."TurnOn", "VISA_in"=w466) -> ("error_out"=w462:errorcluster, "VISA_out"=w463:refnum<visa-resource-name>)  [unwired: 1 in, 1 out]
        n162 = Bundle By Name(cluster=w461, "AC Source Address"=w463) -> (w479:T2)
      }
      frame "RLYInit" {
        # "0xAAAA"
        n163 = Bundle By Name(cluster=w482, "RLY.Num"=T10."AA", "RLY.ON/OFF"=TRUE, "RLY.REST?"=u16 0) -> (w481:T2)
        n164 = Unbundle By Name(w481) -> ("RLY"=w489:T13, "RlyPort"=w494:refnum<visa-resource-name>)
        n165 = VISA Flush I/O Buffer(VISA resource name=w494, error in (no error)=w493) -> (VISA resource name out=w495:refnum<visa-resource-name>, error out=w492:errorcluster)  [unwired: 1 in]
        n166 = call "RLY_Select.vi"("error in"=w492, "RLY"=w489) -> ("error out"=w491:errorcluster, "hex string"=w490:string)
        n167 = VISA Write(VISA resource name=w495, write buffer=w490, error in (no error)=w491) -> (VISA resource name out=w488:refnum<visa-resource-name>, error out=w486:errorcluster)  [unwired: 1 out]
        n168 = Bundle By Name(cluster=w481, "RlyPort"=w488) -> (w487:T2)
      }
      frame "RlyTest1_ON" {
        n169 = Unbundle By Name(w506) -> ("Socket"=w502:enum16{"ABC", "DEF", "GHI"}, "RlyPort"=w507:refnum<visa-resource-name>)
        n170 = case shown="\"GHI\"" w502 {
          tunnel: [T10."11" ("RLY.Num") T10."14" ("RLY.Num") T10."17" ("RLY.Num")] -> w501
          frame "ABC", Default {
            # "A"
          }
          frame "DEF" {
            # "D"
          }
          frame "GHI" {
            # "G"
          }
        }
        n171 = Bundle By Name(cluster=w506, "RLY.Num"=w501, "RLY.ON/OFF"=TRUE) -> (w504:T2)
        n172 = VISA Flush I/O Buffer(VISA resource name=w507, error in (no error)=w510) -> (VISA resource name out=w512:refnum<visa-resource-name>, error out=w509:errorcluster)  [unwired: 1 in]
        n173 = Unbundle By Name(w504) -> ("RLY"=w505:T13)
        n174 = call "RLY_Select.vi"("error in"=w509, "RLY"=w505) -> ("error out"=w508:errorcluster, "hex string"=w511:string)
        n175 = VISA Write(VISA resource name=w512, write buffer=w511, error in (no error)=w508) -> (VISA resource name out=w497:refnum<visa-resource-name>, error out=w500:errorcluster)  [unwired: 1 out]
        n176 = flat-sequence {
          tunnel: w500 -> [w515]
          tunnel: [w515] -> w499
          tunnel: [w514] -> w498
          tunnel: w497 -> [w514]
          frame #0 {
            n177 = Wait (ms)(milliseconds to wait=u32 100) -> ()  [unwired: 1 out]
          }
        }
        n178 = Bundle By Name(cluster=w504, "RlyPort"=w498) -> (w503:T2)
      }
      frame "RlyTest1_OFF" {
        n179 = Unbundle By Name(w529) -> ("Socket"=w525:enum16{"ABC", "DEF", "GHI"}, "RlyPort"=w530:refnum<visa-resource-name>)
        n180 = case shown="\"ABC\", Default" w525 {
          tunnel: [T10."11" ("RLY.Num") T10."14" ("RLY.Num") T10."17" ("RLY.Num")] -> w524
          frame "ABC", Default {
            # "A"
          }
          frame "DEF" {
            # "D"
          }
          frame "GHI" {
            # "G"
          }
        }
        n181 = Bundle By Name(cluster=w529, "RLY.Num"=w524, "RLY.ON/OFF"=FALSE) -> (w527:T2)
        n182 = VISA Flush I/O Buffer(VISA resource name=w530, error in (no error)=w533) -> (VISA resource name out=w535:refnum<visa-resource-name>, error out=w532:errorcluster)  [unwired: 1 in]
        n183 = Unbundle By Name(w527) -> ("RLY"=w528:T13)
        n184 = call "RLY_Select.vi"("error in"=w532, "RLY"=w528) -> ("error out"=w531:errorcluster, "hex string"=w534:string)
        n185 = VISA Write(VISA resource name=w535, write buffer=w534, error in (no error)=w531) -> (VISA resource name out=w520:refnum<visa-resource-name>, error out=w523:errorcluster)  [unwired: 1 out]
        n186 = flat-sequence {
          tunnel: w523 -> [w538]
          tunnel: [w538] -> w522
          tunnel: [w537] -> w521
          tunnel: w520 -> [w537]
          frame #0 {
            n187 = Wait (ms)(milliseconds to wait=u32 100) -> ()  [unwired: 1 out]
          }
        }
        n188 = Bundle By Name(cluster=w527, "RlyPort"=w521) -> (w526:T2)
      }
      frame "RlyWarm1_ON" {
        n189 = Unbundle By Name(w552) -> ("Socket"=w548:enum16{"ABC", "DEF", "GHI"}, "RlyPort"=w553:refnum<visa-resource-name>)
        n190 = case shown="\"ABC\", Default" w548 {
          tunnel: [T10."01" ("RLY.Num") T10."04" ("RLY.Num") T10."07" ("RLY.Num")] -> w547
          frame "ABC", Default {
            # "A"
          }
          frame "DEF" {
            # "D"
          }
          frame "GHI" {
            # "G"
          }
        }
        n191 = Bundle By Name(cluster=w552, "RLY.Num"=w547, "RLY.ON/OFF"=TRUE) -> (w550:T2)
        n192 = VISA Flush I/O Buffer(VISA resource name=w553, error in (no error)=w556) -> (VISA resource name out=w558:refnum<visa-resource-name>, error out=w555:errorcluster)  [unwired: 1 in]
        n193 = Unbundle By Name(w550) -> ("RLY"=w551:T13)
        n194 = call "RLY_Select.vi"("error in"=w555, "RLY"=w551) -> ("error out"=w554:errorcluster, "hex string"=w557:string)
        n195 = VISA Write(VISA resource name=w558, write buffer=w557, error in (no error)=w554) -> (VISA resource name out=w543:refnum<visa-resource-name>, error out=w546:errorcluster)  [unwired: 1 out]
        n196 = flat-sequence {
          tunnel: w546 -> [w561]
          tunnel: [w561] -> w545
          tunnel: [w560] -> w544
          tunnel: w543 -> [w560]
          frame #0 {
            n197 = Wait (ms)(milliseconds to wait=u32 100) -> ()  [unwired: 1 out]
          }
        }
        n198 = Bundle By Name(cluster=w550, "RlyPort"=w544) -> (w549:T2)
      }
      frame "RlyWarm1_OFF" {
        n199 = Unbundle By Name(w575) -> ("Socket"=w571:enum16{"ABC", "DEF", "GHI"}, "RlyPort"=w576:refnum<visa-resource-name>)
        n200 = case shown="\"ABC\", Default" w571 {
          tunnel: [T10."01" ("RLY.Num") T10."04" ("RLY.Num") T10."07" ("RLY.Num")] -> w570
          frame "ABC", Default {
            # "A"
          }
          frame "DEF" {
            # "D"
          }
          frame "GHI" {
            # "G"
          }
        }
        n201 = Bundle By Name(cluster=w575, "RLY.Num"=w570, "RLY.ON/OFF"=FALSE) -> (w573:T2)
        n202 = VISA Flush I/O Buffer(VISA resource name=w576, error in (no error)=w579) -> (VISA resource name out=w581:refnum<visa-resource-name>, error out=w578:errorcluster)  [unwired: 1 in]
        n203 = Unbundle By Name(w573) -> ("RLY"=w574:T13)
        n204 = call "RLY_Select.vi"("error in"=w578, "RLY"=w574) -> ("error out"=w577:errorcluster, "hex string"=w580:string)
        n205 = VISA Write(VISA resource name=w581, write buffer=w580, error in (no error)=w577) -> (VISA resource name out=w566:refnum<visa-resource-name>, error out=w569:errorcluster)  [unwired: 1 out]
        n206 = flat-sequence {
          tunnel: w569 -> [w584]
          tunnel: [w584] -> w568
          tunnel: [w583] -> w567
          tunnel: w566 -> [w583]
          frame #0 {
            n207 = Wait (ms)(milliseconds to wait=u32 100) -> ()  [unwired: 1 out]
          }
        }
        n208 = Bundle By Name(cluster=w573, "RlyPort"=w567) -> (w572:T2)
      }
      frame "RlyTest2_ON" {
        n209 = Unbundle By Name(w598) -> ("Socket"=w594:enum16{"ABC", "DEF", "GHI"}, "RlyPort"=w599:refnum<visa-resource-name>)
        n210 = case shown="\"GHI\"" w594 {
          tunnel: [T10."12" ("RLY.Num") T10."15" ("RLY.Num") T10."18" ("RLY.Num")] -> w593
          frame "ABC", Default {
            # "B"
          }
          frame "DEF" {
            # "E"
          }
          frame "GHI" {
            # "H"
          }
        }
        n211 = Bundle By Name(cluster=w598, "RLY.Num"=w593, "RLY.ON/OFF"=TRUE) -> (w596:T2)
        n212 = VISA Flush I/O Buffer(VISA resource name=w599, error in (no error)=w602) -> (VISA resource name out=w604:refnum<visa-resource-name>, error out=w601:errorcluster)  [unwired: 1 in]
        n213 = Unbundle By Name(w596) -> ("RLY"=w597:T13)
        n214 = call "RLY_Select.vi"("error in"=w601, "RLY"=w597) -> ("error out"=w600:errorcluster, "hex string"=w603:string)
        n215 = VISA Write(VISA resource name=w604, write buffer=w603, error in (no error)=w600) -> (VISA resource name out=w589:refnum<visa-resource-name>, error out=w592:errorcluster)  [unwired: 1 out]
        n216 = flat-sequence {
          tunnel: w592 -> [w607]
          tunnel: [w607] -> w591
          tunnel: [w606] -> w590
          tunnel: w589 -> [w606]
          frame #0 {
            n217 = Wait (ms)(milliseconds to wait=u32 100) -> ()  [unwired: 1 out]
          }
        }
        n218 = Bundle By Name(cluster=w596, "RlyPort"=w590) -> (w595:T2)
      }
      frame "RlyTest2_OFF" {
        n219 = Unbundle By Name(w621) -> ("Socket"=w617:enum16{"ABC", "DEF", "GHI"}, "RlyPort"=w622:refnum<visa-resource-name>)
        n220 = case shown="\"ABC\", Default" w617 {
          tunnel: [T10."12" ("RLY.Num") T10."15" ("RLY.Num") T10."18" ("RLY.Num")] -> w616
          frame "ABC", Default {
            # "B"
          }
          frame "DEF" {
            # "E"
          }
          frame "GHI" {
            # "H"
          }
        }
        n221 = Bundle By Name(cluster=w621, "RLY.Num"=w616, "RLY.ON/OFF"=FALSE) -> (w619:T2)
        n222 = VISA Flush I/O Buffer(VISA resource name=w622, error in (no error)=w625) -> (VISA resource name out=w627:refnum<visa-resource-name>, error out=w624:errorcluster)  [unwired: 1 in]
        n223 = Unbundle By Name(w619) -> ("RLY"=w620:T13)
        n224 = call "RLY_Select.vi"("error in"=w624, "RLY"=w620) -> ("error out"=w623:errorcluster, "hex string"=w626:string)
        n225 = VISA Write(VISA resource name=w627, write buffer=w626, error in (no error)=w623) -> (VISA resource name out=w612:refnum<visa-resource-name>, error out=w615:errorcluster)  [unwired: 1 out]
        n226 = flat-sequence {
          tunnel: w615 -> [w630]
          tunnel: [w630] -> w614
          tunnel: [w629] -> w613
          tunnel: w612 -> [w629]
          frame #0 {
            n227 = Wait (ms)(milliseconds to wait=u32 100) -> ()  [unwired: 1 out]
          }
        }
        n228 = Bundle By Name(cluster=w619, "RlyPort"=w613) -> (w618:T2)
      }
      frame "RlyWarm2_ON" {
        n229 = Unbundle By Name(w644) -> ("Socket"=w640:enum16{"ABC", "DEF", "GHI"}, "RlyPort"=w645:refnum<visa-resource-name>)
        n230 = case shown="\"ABC\", Default" w640 {
          tunnel: [T10."02" ("RLY.Num") T10."05" ("RLY.Num") T10."08" ("RLY.Num")] -> w639
          frame "ABC", Default {
            # "B"
          }
          frame "DEF" {
            # "E"
          }
          frame "GHI" {
            # "H"
          }
        }
        n231 = Bundle By Name(cluster=w644, "RLY.Num"=w639, "RLY.ON/OFF"=TRUE) -> (w642:T2)
        n232 = VISA Flush I/O Buffer(VISA resource name=w645, error in (no error)=w648) -> (VISA resource name out=w650:refnum<visa-resource-name>, error out=w647:errorcluster)  [unwired: 1 in]
        n233 = Unbundle By Name(w642) -> ("RLY"=w643:T13)
        n234 = call "RLY_Select.vi"("error in"=w647, "RLY"=w643) -> ("error out"=w646:errorcluster, "hex string"=w649:string)
        n235 = VISA Write(VISA resource name=w650, write buffer=w649, error in (no error)=w646) -> (VISA resource name out=w635:refnum<visa-resource-name>, error out=w638:errorcluster)  [unwired: 1 out]
        n236 = flat-sequence {
          tunnel: w638 -> [w653]
          tunnel: [w653] -> w637
          tunnel: [w652] -> w636
          tunnel: w635 -> [w652]
          frame #0 {
            n237 = Wait (ms)(milliseconds to wait=u32 100) -> ()  [unwired: 1 out]
          }
        }
        n238 = Bundle By Name(cluster=w642, "RlyPort"=w636) -> (w641:T2)
      }
      frame "RlyWarm2_OFF" {
        n239 = Unbundle By Name(w667) -> ("Socket"=w663:enum16{"ABC", "DEF", "GHI"}, "RlyPort"=w668:refnum<visa-resource-name>)
        n240 = case shown="\"ABC\", Default" w663 {
          tunnel: [T10."02" ("RLY.Num") T10."05" ("RLY.Num") T10."08" ("RLY.Num")] -> w662
          frame "ABC", Default {
            # "B"
          }
          frame "DEF" {
            # "E"
          }
          frame "GHI" {
            # "H"
          }
        }
        n241 = Bundle By Name(cluster=w667, "RLY.Num"=w662, "RLY.ON/OFF"=FALSE) -> (w665:T2)
        n242 = VISA Flush I/O Buffer(VISA resource name=w668, error in (no error)=w671) -> (VISA resource name out=w673:refnum<visa-resource-name>, error out=w670:errorcluster)  [unwired: 1 in]
        n243 = Unbundle By Name(w665) -> ("RLY"=w666:T13)
        n244 = call "RLY_Select.vi"("error in"=w670, "RLY"=w666) -> ("error out"=w669:errorcluster, "hex string"=w672:string)
        n245 = VISA Write(VISA resource name=w673, write buffer=w672, error in (no error)=w669) -> (VISA resource name out=w658:refnum<visa-resource-name>, error out=w661:errorcluster)  [unwired: 1 out]
        n246 = flat-sequence {
          tunnel: w661 -> [w676]
          tunnel: [w676] -> w660
          tunnel: [w675] -> w659
          tunnel: w658 -> [w675]
          frame #0 {
            n247 = Wait (ms)(milliseconds to wait=u32 100) -> ()  [unwired: 1 out]
          }
        }
        n248 = Bundle By Name(cluster=w665, "RlyPort"=w659) -> (w664:T2)
      }
      frame "RlyTest3_ON" {
        n249 = Unbundle By Name(w690) -> ("Socket"=w686:enum16{"ABC", "DEF", "GHI"}, "RlyPort"=w691:refnum<visa-resource-name>)
        n250 = case shown="\"ABC\", Default" w686 {
          tunnel: [T10."13" ("RLY.Num") T10."16" ("RLY.Num") T10."19" ("RLY.Num")] -> w685
          frame "ABC", Default {
            # "C"
          }
          frame "DEF" {
            # "F"
          }
          frame "GHI" {
            # "I"
          }
        }
        n251 = Bundle By Name(cluster=w690, "RLY.Num"=w685, "RLY.ON/OFF"=TRUE) -> (w688:T2)
        n252 = VISA Flush I/O Buffer(VISA resource name=w691, error in (no error)=w694) -> (VISA resource name out=w696:refnum<visa-resource-name>, error out=w693:errorcluster)  [unwired: 1 in]
        n253 = Unbundle By Name(w688) -> ("RLY"=w689:T13)
        n254 = call "RLY_Select.vi"("error in"=w693, "RLY"=w689) -> ("error out"=w692:errorcluster, "hex string"=w695:string)
        n255 = VISA Write(VISA resource name=w696, write buffer=w695, error in (no error)=w692) -> (VISA resource name out=w681:refnum<visa-resource-name>, error out=w684:errorcluster)  [unwired: 1 out]
        n256 = flat-sequence {
          tunnel: w684 -> [w699]
          tunnel: [w699] -> w683
          tunnel: [w698] -> w682
          tunnel: w681 -> [w698]
          frame #0 {
            n257 = Wait (ms)(milliseconds to wait=u32 100) -> ()  [unwired: 1 out]
          }
        }
        n258 = Bundle By Name(cluster=w688, "RlyPort"=w682) -> (w687:T2)
      }
      frame "RlyTest3_OFF" {
        n259 = Unbundle By Name(w713) -> ("Socket"=w709:enum16{"ABC", "DEF", "GHI"}, "RlyPort"=w714:refnum<visa-resource-name>)
        n260 = case shown="\"ABC\", Default" w709 {
          tunnel: [T10."13" ("RLY.Num") T10."16" ("RLY.Num") T10."19" ("RLY.Num")] -> w708
          frame "ABC", Default {
            # "C"
          }
          frame "DEF" {
            # "F"
          }
          frame "GHI" {
            # "I"
          }
        }
        n261 = Bundle By Name(cluster=w713, "RLY.Num"=w708, "RLY.ON/OFF"=FALSE) -> (w711:T2)
        n262 = VISA Flush I/O Buffer(VISA resource name=w714, error in (no error)=w717) -> (VISA resource name out=w719:refnum<visa-resource-name>, error out=w716:errorcluster)  [unwired: 1 in]
        n263 = Unbundle By Name(w711) -> ("RLY"=w712:T13)
        n264 = call "RLY_Select.vi"("error in"=w716, "RLY"=w712) -> ("error out"=w715:errorcluster, "hex string"=w718:string)
        n265 = VISA Write(VISA resource name=w719, write buffer=w718, error in (no error)=w715) -> (VISA resource name out=w704:refnum<visa-resource-name>, error out=w707:errorcluster)  [unwired: 1 out]
        n266 = flat-sequence {
          tunnel: w707 -> [w722]
          tunnel: [w722] -> w706
          tunnel: [w721] -> w705
          tunnel: w704 -> [w721]
          frame #0 {
            n267 = Wait (ms)(milliseconds to wait=u32 100) -> ()  [unwired: 1 out]
          }
        }
        n268 = Bundle By Name(cluster=w711, "RlyPort"=w705) -> (w710:T2)
      }
      frame "RlyWarm3_ON" {
        n269 = Unbundle By Name(w736) -> ("Socket"=w732:enum16{"ABC", "DEF", "GHI"}, "RlyPort"=w737:refnum<visa-resource-name>)
        n270 = case shown="\"ABC\", Default" w732 {
          tunnel: [T10."03" ("RLY.Num") T10."06" ("RLY.Num") T10."09" ("RLY.Num")] -> w731
          frame "ABC", Default {
            # "C"
          }
          frame "DEF" {
            # "F"
          }
          frame "GHI" {
            # "I"
          }
        }
        n271 = Bundle By Name(cluster=w736, "RLY.Num"=w731, "RLY.ON/OFF"=TRUE) -> (w734:T2)
        n272 = VISA Flush I/O Buffer(VISA resource name=w737, error in (no error)=w740) -> (VISA resource name out=w742:refnum<visa-resource-name>, error out=w739:errorcluster)  [unwired: 1 in]
        n273 = Unbundle By Name(w734) -> ("RLY"=w735:T13)
        n274 = call "RLY_Select.vi"("error in"=w739, "RLY"=w735) -> ("error out"=w738:errorcluster, "hex string"=w741:string)
        n275 = VISA Write(VISA resource name=w742, write buffer=w741, error in (no error)=w738) -> (VISA resource name out=w727:refnum<visa-resource-name>, error out=w730:errorcluster)  [unwired: 1 out]
        n276 = flat-sequence {
          tunnel: w730 -> [w745]
          tunnel: [w745] -> w729
          tunnel: [w744] -> w728
          tunnel: w727 -> [w744]
          frame #0 {
            n277 = Wait (ms)(milliseconds to wait=u32 100) -> ()  [unwired: 1 out]
          }
        }
        n278 = Bundle By Name(cluster=w734, "RlyPort"=w728) -> (w733:T2)
      }
      frame "RlyWarm3_OFF" {
        n279 = Unbundle By Name(w759) -> ("Socket"=w755:enum16{"ABC", "DEF", "GHI"}, "RlyPort"=w760:refnum<visa-resource-name>)
        n280 = case shown="\"ABC\", Default" w755 {
          tunnel: [T10."03" ("RLY.Num") T10."06" ("RLY.Num") T10."09" ("RLY.Num")] -> w754
          frame "ABC", Default {
            # "C"
          }
          frame "DEF" {
            # "F"
          }
          frame "GHI" {
            # "I"
          }
        }
        n281 = Bundle By Name(cluster=w759, "RLY.Num"=w754, "RLY.ON/OFF"=FALSE) -> (w757:T2)
        n282 = VISA Flush I/O Buffer(VISA resource name=w760, error in (no error)=w763) -> (VISA resource name out=w765:refnum<visa-resource-name>, error out=w762:errorcluster)  [unwired: 1 in]
        n283 = Unbundle By Name(w757) -> ("RLY"=w758:T13)
        n284 = call "RLY_Select.vi"("error in"=w762, "RLY"=w758) -> ("error out"=w761:errorcluster, "hex string"=w764:string)
        n285 = VISA Write(VISA resource name=w765, write buffer=w764, error in (no error)=w761) -> (VISA resource name out=w750:refnum<visa-resource-name>, error out=w753:errorcluster)  [unwired: 1 out]
        n286 = flat-sequence {
          tunnel: w753 -> [w768]
          tunnel: [w768] -> w752
          tunnel: [w767] -> w751
          tunnel: w750 -> [w767]
          frame #0 {
            n287 = Wait (ms)(milliseconds to wait=u32 100) -> ()  [unwired: 1 out]
          }
        }
        n288 = Bundle By Name(cluster=w757, "RlyPort"=w751) -> (w756:T2)
      }
      frame "RlyLoad_ON" {
        n289 = Unbundle By Name(w782) -> ("Socket"=w778:enum16{"ABC", "DEF", "GHI"}, "RlyPort"=w783:refnum<visa-resource-name>)
        n290 = case shown="\"ABC\", Default" w778 {
          tunnel: [T10."21" ("RLY.Num") T10."22" ("RLY.Num") T10."23" ("RLY.Num")] -> w777
          frame "ABC", Default {
            # "ABC"
          }
          frame "DEF" {
            # "DEF"
          }
          frame "GHI" {
            # "GHI"
          }
        }
        n291 = Bundle By Name(cluster=w782, "RLY.Num"=w777, "RLY.ON/OFF"=TRUE) -> (w780:T2)
        n292 = VISA Flush I/O Buffer(VISA resource name=w783, error in (no error)=w786) -> (VISA resource name out=w788:refnum<visa-resource-name>, error out=w785:errorcluster)  [unwired: 1 in]
        n293 = Unbundle By Name(w780) -> ("RLY"=w781:T13)
        n294 = call "RLY_Select.vi"("error in"=w785, "RLY"=w781) -> ("error out"=w784:errorcluster, "hex string"=w787:string)
        n295 = VISA Write(VISA resource name=w788, write buffer=w787, error in (no error)=w784) -> (VISA resource name out=w773:refnum<visa-resource-name>, error out=w776:errorcluster)  [unwired: 1 out]
        n296 = flat-sequence {
          tunnel: w776 -> [w791]
          tunnel: [w791] -> w775
          tunnel: [w790] -> w774
          tunnel: w773 -> [w790]
          frame #0 {
            n297 = Wait (ms)(milliseconds to wait=u32 100) -> ()  [unwired: 1 out]
          }
        }
        n298 = Bundle By Name(cluster=w780, "RlyPort"=w774) -> (w779:T2)
      }
      frame "RlyLoad_OFF" {
        n299 = Unbundle By Name(w805) -> ("Socket"=w801:enum16{"ABC", "DEF", "GHI"}, "RlyPort"=w806:refnum<visa-resource-name>)
        n300 = case shown="\"ABC\", Default" w801 {
          tunnel: [T10."21" ("RLY.Num") T10."22" ("RLY.Num") T10."23" ("RLY.Num")] -> w800
          frame "ABC", Default {
            # "ABC"
          }
          frame "DEF" {
            # "DEF"
          }
          frame "GHI" {
            # "GHI"
          }
        }
        n301 = Bundle By Name(cluster=w805, "RLY.Num"=w800, "RLY.ON/OFF"=FALSE) -> (w803:T2)
        n302 = VISA Flush I/O Buffer(VISA resource name=w806, error in (no error)=w809) -> (VISA resource name out=w811:refnum<visa-resource-name>, error out=w808:errorcluster)  [unwired: 1 in]
        n303 = Unbundle By Name(w803) -> ("RLY"=w804:T13)
        n304 = call "RLY_Select.vi"("error in"=w808, "RLY"=w804) -> ("error out"=w807:errorcluster, "hex string"=w810:string)
        n305 = VISA Write(VISA resource name=w811, write buffer=w810, error in (no error)=w807) -> (VISA resource name out=w796:refnum<visa-resource-name>, error out=w799:errorcluster)  [unwired: 1 out]
        n306 = flat-sequence {
          tunnel: w799 -> [w814]
          tunnel: [w814] -> w798
          tunnel: [w813] -> w797
          tunnel: w796 -> [w813]
          frame #0 {
            n307 = Wait (ms)(milliseconds to wait=u32 100) -> ()  [unwired: 1 out]
          }
        }
        n308 = Bundle By Name(cluster=w803, "RlyPort"=w797) -> (w802:T2)
      }
      frame "UISet1" {
        w818 = TRUE ("Load (F:Off)")
        n309 = Bundle By Name(cluster=w832, "Step.PM"=string[] ["PMUpdate", "GetInputU", "GetInputI", "GetInputP", "CalcuateP.F", "Integrate", "PM2UI_1"] ("StepName")) -> (w830:T2)
        n310 = Bundle By Name(cluster=w830, "Load.Record"=w818, "Load.Load (ON/Off)"=w818, "Load.Index"=0, "Load.Current Level (F:Low)"=u16 0, "Step.Load"=string[] ["LoadUpdate", "LoadMode", "SetLoad ", "LoadRead", "Load2UI_1"]) -> (w826:T2)
        n311 = Bundle By Name(cluster=w826, "Message"="#1_100%Testing", "Step.UI"=string[] ["RlyWarm1_OFF", "Rly_Test1_ON", "SetAC", "UpdatePM", "UpdateLoad"]) -> (w825:T2)
        n312 = call-poly "Enqueue Message.vi"("error in (no error)"=w823, "Message"="UPdateUI", "Message Queue"=w821) -> ("error out"=w822:errorcluster)  [unwired: 7 in, 1 out]
      }
      frame "UISet2" {
        w833 = TRUE ("Load (F:Off)")
        n313 = Bundle By Name(cluster=w847, "Step.PM"=string[] ["GetInputU", "GetInputI", "GetInputP", "CalcuateP.F", "Integrate", "PM2UI"] ("StepName")) -> (w845:T2)
        n314 = Bundle By Name(cluster=w845, "Load.Record"=w833, "Load.Load (ON/Off)"=w833, "Load.Index"=0, "Load.Current Level (F:Low)"=u16 0, "Step.Load"=string[] ["LoadMode", "SetLoad ", "LoadRead", "Load2UI_2"]) -> (w841:T2)
        n315 = Bundle By Name(cluster=w841, "Message"="#2_100%Testing", "Step.UI"=string[] ["RlWarm2_OFF", "Rly_Test1_OFF", "Rly_Test2_ON", "UpdatePM", "UpdateLoad"]) -> (w840:T2)
        n316 = call-poly "Enqueue Message.vi"("error in (no error)"=w838, "Message"="UPdateUI", "Message Queue"=w836) -> ("error out"=w837:errorcluster)  [unwired: 7 in, 1 out]
      }
      frame "UISet3" {
        w848 = TRUE ("Load (F:Off)")
        n317 = Bundle By Name(cluster=w862, "Step.PM"=string[] ["GetInputU", "GetInputI", "GetInputP", "CalcuateP.F", "Integrate", "PM2UI"] ("StepName")) -> (w860:T2)
        n318 = Bundle By Name(cluster=w860, "Load.Record"=w848, "Load.Load (ON/Off)"=w848, "Load.Index"=0, "Load.Current Level (F:Low)"=u16 0, "Step.Load"=string[] ["LoadMode", "SetLoad ", "LoadRead", "Load2UI_3"]) -> (w856:T2)
        n319 = Bundle By Name(cluster=w856, "Message"="#3_100%Testing", "Step.UI"=string[] ["RlWarm3_OFF", "Rly_Test2_OFF", "Rly_Test3_ON", "UpdatePM", "UpdateLoad"]) -> (w855:T2)
        n320 = call-poly "Enqueue Message.vi"("error in (no error)"=w853, "Message"="UPdateUI", "Message Queue"=w851) -> ("error out"=w852:errorcluster)  [unwired: 7 in, 1 out]
      }
      frame "UpdateUI" {
        # "Update Display - Convert the message data to a string to display in the Data Display indicator."
        n321 = Unbundle By Name(w866) -> ("Message"=→"Status":string, "Step.UI"=w864:string[])
        n322 = call-poly "Enqueue Message.vi"("error in (no error)"=w867, "Message Array"=w864, "Message Queue"=w868) -> ("error out"=w863:errorcluster)  [unwired: 7 in, 1 out]
      }
      frame "UpdatePM" {
        # "Update Display - Convert the message data to a string to display in the Data Display indicator."
        n323 = Unbundle By Name(w871) -> ("Step.PM"=w874:string[], "InputData"=w870:T6)
        n324 = Build Array(w870) -> (w869:T14)
        n325 = call-poly "Enqueue Message.vi"("error in (no error)"=w875, "Message Data Array"=w869, "Message Array"=w874, "Message Queue"=w873) -> ("error out"=w872:errorcluster)  [unwired: 6 in, 1 out]
      }
      frame "UpdateLoad" {
        # "Update Display - Convert the message data to a string to display in the Data Display indicator."
        n326 = Unbundle By Name(w876) -> ("Step.Load"=w881:string[], "Load"=w877:T4)
        n327 = Build Array(w877) -> (w878:T5)
        n328 = call-poly "Enqueue Message.vi"("error in (no error)"=w882, "Message Data Array"=w878, "Message Array"=w881, "Message Queue"=w880) -> ("error out"=w879:errorcluster)  [unwired: 6 in, 1 out]
      }
      frame "LoadDataUpdate" {
        n329 = Variant To Data(error in=w888, type=T4 {"Current Level (F:Low)"=0, "OutputLoad[]"=[], "Index"=0, "Load (ON/Off)"=FALSE, "Channel (0:Channel 1)"=0, "Value[]"={"A"=[], "W"=[], "V"=[]}, "Record"=FALSE} ("Load"), Variant=w886) -> (data=w883:T4, error out=w887:errorcluster)
        n330 = Bundle By Name(cluster=w885, "Load"=w883) -> (w884:T2)
      }
      frame "PMDataUpdate" {
        n331 = Variant To Data(error in=w895, type=T4 {"Current Level (F:Low)"=0, "OutputLoad[]"=[], "Index"=0, "Load (ON/Off)"=FALSE, "Channel (0:Channel 1)"=0, "Value[]"={"A"=[], "W"=[], "V"=[]}, "Record"=FALSE} ("Load"), Variant=w893) -> (data=w890:T4, error out=w894:errorcluster)
        n332 = Bundle By Name(cluster=w892, "Load"=w890) -> (w891:T2)
      }
      frame "Counter" {
        # "30mins"
        n333 = Unbundle By Name(w906) -> ("WarmUp Time"=w897:dbl)
        n334 = Increment(x=w897) -> (x+1=w905:dbl)
        n335 = call "Elapsed Time"("Time Target (s)"=w897, "error in (no error)"=w899) -> ("Elapsed Time (s)"=w904:dbl, "error out"=w898:errorcluster)  [unwired: 10 in, 6 out]
        n336 = Subtract(x=w905, y=w904) -> (x-y=w902:dbl)
        n337 = Format Date/Time String(time format string (%c)="%M:%S", seconds (now)=w902, UTC format=TRUE) -> (date/time string=→"Counter":string)
      }
      frame "Error" {
        # "Error - Display an error dialog. This message is sent by the \"Error Handler\" VIs at the end of other loops in this application."
        n338 = Variant To Data(error in=w913, type=errorcluster {"status"=FALSE, "code"=0, "source"=""} ("error constant"), Variant=w911) -> (data=w909:errorcluster, error out=w908:errorcluster)
        n339 = call <vilib>:"Simple Error Handler.vi"("error in (no error)"=w909) -> ()  [unwired: 4 in, 5 out]
        n340 = Merge Errors(w908) -> (w907:errorcluster)
      }
      frame "Confirm Quit" {
        # "Confirm Quit - Message that can confirm whether or not the user wants to exit the application."
        n341 = call-poly "Enqueue Message.vi"("Priority Message? (F)"=TRUE, "error in (no error)"=w920, "Message"="Exit", "Message Queue"=w916) -> ("error out"=w917:errorcluster)  [unwired: 6 in, 1 out]
        n342 = Merge Errors(w917) -> (w918:errorcluster)
      }
      frame "---Copy This Frame---" {
        # "Duplicate this frame when creating new messages.  Change this comment in the duplicated frame to describe this message."
        n343 = Merge Errors(w923) -> (w921:errorcluster)
      }
      frame "Exit" {
        # "Stop the VI"
        # "Release the message queue reference"
        # "Exit - Exit the application."
        n344 = Variant To Data(type=errorcluster {"status"=FALSE, "code"=0, "source"=""} ("error constant"), Variant=w924) -> (data=w925:errorcluster)  [unwired: 1 in, 1 out]
        n345 = call <vilib>:"Simple Error Handler.vi"("error in (no error)"=w925) -> ()  [unwired: 4 in, 5 out]
        n346 = call "Fire User Event - Stop.vi"("User Event - Stop"=w929) -> ("error out"=w928:errorcluster)  [unwired: 10 in]
        n347 = Release Queue(queue=w934, error in (no error)=w927) -> (error out=w931:errorcluster)  [unwired: 1 in, 2 out]
        n348 = Merge Errors(w928, w931) -> (w930:errorcluster)
      }
      frame "message" {
        # "'Default' case only runs if there is a message that isn't defined in any of the other cases.  Output a programming error."
        n349 = xnode "Error Ring"("parameter 0"=w935) -> ("error out"=w936:errorcluster)
      }
    }
    n350 = call "Error Handler - Message Handling Loop.vi"("error in (no error)"=w372, "Message Queue"=w374) -> ("dup error in"=w373:errorcluster)  [unwired: 8 in, 1 out]
  }
  n351 = while {
    tunnel: w5 -> [w951]
    shift-right: [w949] -> w13
    shift-left: w10 -> [w950]
    tunnel: [w945] -> w11
    stop <- w947 stop-if-true
    # "Event Handling Loop"
    n352 = event shown="[0] \"Do Something <Replace Me>\": Value Change" {
      selector: w950 -> [_ _ _ _ _ _]
      dyn-events: [_ _ _ _ _ _] -> w949
      timeout: _ -> [_ _ _ _ _ _]
      tunnel: [_ _ _ _ _ TRUE ("Discard?")] -> w947
      tunnel: w951 -> [w955 w959 w964 w966 w971 w974]
      tunnel: [w952 w956 w963 _ w970 _] -> w948
      tunnel: [w954 w958 w962 w966 w969 w974] -> w946
      event "Do Something <Replace Me>": Value Change {
        n353 = event-data() -> ()  [unwired: 1 in, 1 out]
        n354 = call-poly "Enqueue Message.vi"("Message"="Something", "Message Queue"=w955) -> ("error out"=w952:errorcluster, "dup Message Queue"=w954:refnum<queue>)  [unwired: 8 in]
      }
      event "Do Something Else <Replace Me>": Value Change {
        # "#CodeNeeded - Send the appropriate message for this user interface event."
        n355 = event-data() -> ()  [unwired: 1 in, 1 out]
        n356 = call-poly "Enqueue Message.vi"("Message"="Something Else", "Message Queue"=w959) -> ("error out"=w956:errorcluster, "dup Message Queue"=w958:refnum<queue>)  [unwired: 8 in]
      }
      event Panel Close? {
        # "Send the 'Confirm Quit' message if the user closes the panel of the VI. Discard the event so the 'Confirm Quit' message has a chance to run."
        n357 = event-data() -> ()  [unwired: 1 in, 1 out]
        n358 = call-poly "Enqueue Message.vi"("Priority Message? (F)"=TRUE, "Message"="Confirm Quit", "Message Queue"=w964) -> ("error out"=w963:errorcluster, "dup Message Queue"=w962:refnum<queue>)  [unwired: 7 in]
        n359 = event-data("Discard?"=TRUE) -> ()  [unwired: 1 in, 1 out]
      }
      event Application Instance Close {
        # "#CodeRecommended - When a project closes, all VIs within that project are aborted and leave memory. However, any code placed in this event frame is guaranteed to run to completion, so add any cleanup code that absolutely must happen here."
        n360 = event-data() -> ()  [unwired: 1 in, 1 out]
      }
      event "Exit": Value Change {
        n361 = event-data() -> ()  [unwired: 1 in, 1 out]
        n362 = call-poly "Enqueue Message.vi"("Priority Message? (F)"=TRUE, "Message"="Exit", "Message Queue"=w971) -> ("error out"=w970:errorcluster, "dup Message Queue"=w969:refnum<queue>)  [unwired: 7 in]
      }
      event User Event {
        # "The Message Handling Loop processed an \"Exit\" message, which fired this event to stop the Event Handling Loop."
        n363 = event-data() -> ()  [unwired: 1 in, 1 out]
        n364 = local write "Status"("\"Exit\" button pressed" ("VI Stopped")) -> ()
      }
    }
    n365 = call "Error Handler - Event Handling Loop.vi"("error in (no error)"=w948, "Message Queue"=w946) -> ("dup error in"=w945:errorcluster)  [unwired: 8 in, 1 out]
  }
  n366 = Unregister For Events(event registration refnum=w13, error in=w11) -> (error out=w14:errorcluster)
  n367 = Merge Errors(w14, w17, w7, w1) -> (w15:errorcluster)
  n368 = call "Destroy User Event - Stop.vi"("error in (no error)"=w15, "User Event - Stop"=w9) -> ("error out"=w12:errorcluster)  [unwired: 9 in]
  n369 = disable-structure shown="RUN_TIME_ENGINE==True" {
    disable-tunnel: w12 -> [_ _]
    frame condition #0 (active) {
    }
    frame condition #1 {
      # "Call Quit LabVIEW if running as a built application."
      n370 = Quit LabVIEW() -> ()  [unwired: 1 in]
    }
  }
